vi "CSM_Curve Editor.vi"() -> ()   [LabVIEW 2020, in "Curve Editor.lvlib"]
uses:
  Curve Editor.lvlib
  User Data--cluster.ctl
  <vilib>/Utility/miscctls.llb/LVPointTypeDef.ctl
  7b0969bd-7955-4222-98c9-53128525ee30.vi
  183b1dfd-394f-40bc-8548-5665fe87f6d3.vi
  54737b30-700e-483c-a5e2-87d6bca6278c.vi
  <userlib>/_NEVSTOP/Communicable State Machine(CSM)/AdvanceAPI/CSM - Revert Arguments-Safe String.vi
  <userlib>/_NEVSTOP/Communicable State Machine(CSM)/_Shared/Trim Single-line Text.vi
  <userlib>/_NEVSTOP/Communicable State Machine(CSM)/AdvanceAPI/CSM - Make String Arguments Safe.vi
  <userlib>/_NEVSTOP/Communicable State Machine(CSM)/AdvanceAPI/CSM - Break Down Multiple States String.vi
  <userlib>/_NEVSTOP/Communicable State Machine(CSM)/AdvanceAPI/CSM - Compact Multiple States.vi
  <userlib>/_NEVSTOP/Communicable State Machine(CSM)/AdvanceAPI/CSM - Keywords.vi
  <userlib>/_NEVSTOP/Communicable State Machine(CSM)/addons/API-String-Arugments-Support/_Support/Data To API String Arguments.vi
  <vilib>/Utility/file.llb/Read Delimited Spreadsheet (string).vi
  <userlib>/_NEVSTOP/Communicable State Machine(CSM)/addons/API-String-Arugments-Support/_Support/Convert API String Arguments to Data(variant).vi
  <userlib>/_NEVSTOP/Communicable State Machine(CSM)/Communicable State Machine.lvlib
panel:
  in  "Tab Control":enum32{"Page 1"}(tab)
  in  "动作列表框":i32(listbox) caption="曲线片段"
  in  "循环树形":string(tree) caption="循环编辑"
  in  "打开按钮":bool
  in  "保存按钮":bool
  in  "另存为按钮":bool
  in  "新建按钮":bool
  out "曲线预览":cluster{"X":dbl[], "Y":dbl[]}(graph)
  out "总时长[秒]":dbl format="%.2f"
  out "State History":string
  in  "Name (\"\" to Use UUID)":string="Curve Editor"
  # "曲线编辑"
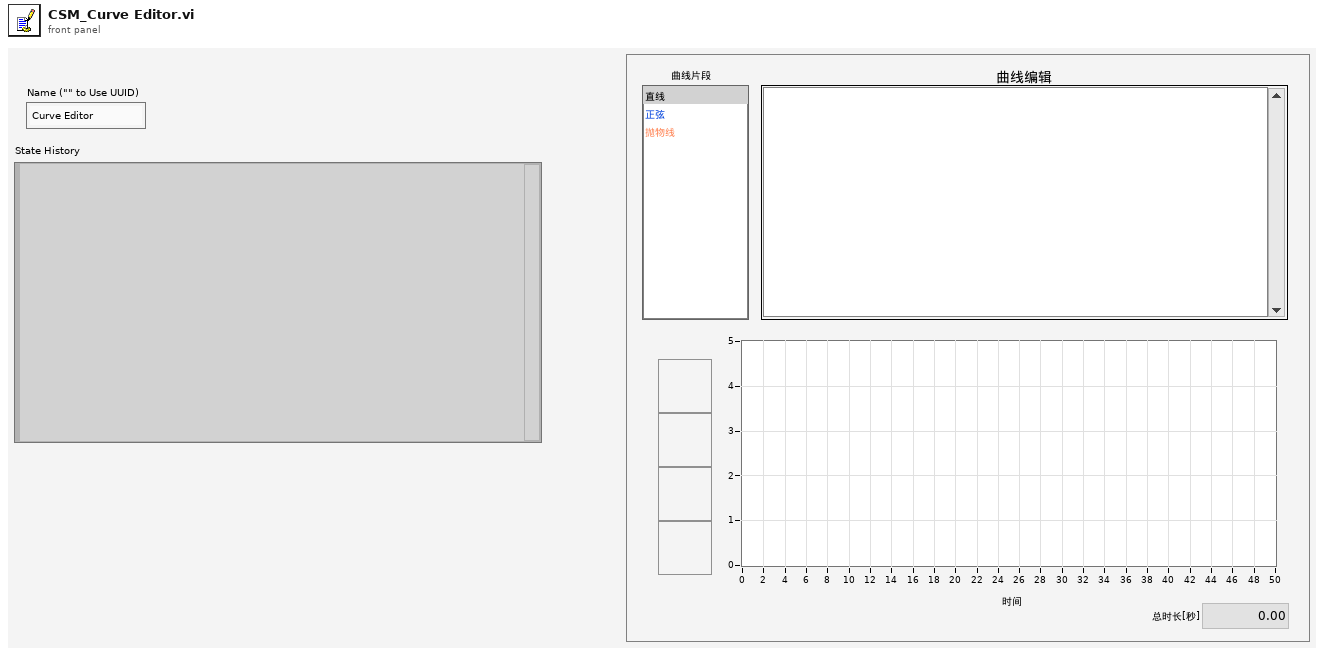
[diagram p1: front panel]
types:
  T1 = enum32{"Invalid", "Standard", "Closed", "Hidden", "Minimized", "Maximized"}
  T2 = enum32{"invalid app kind", "Development System", "Run Time System", "Student Edition", "Embedded LabVIEW", "Evaluation", "Custom"}
  T3 = cluster{"开始路径":path, "默认名称":string, "类型(后缀名)":string, "类型标签":string}
  T4 = typedef "LVPointTypeDef.ctl" = cluster{"Horizontal":i16, "Vertical":i16}
  T5 = enum16{"open", "replace", "create", "open or create", "replace or create", "replace or create with confirmation"}
  T6 = typedef "Communicable State Machine.lvlib/_CSM_Response Source Message.ctl" = cluster{"‘State":string, "’Arguments":string, "’Error":errorcluster}
  T7 = typedef "LVPoint32TypeDef.ctl" = cluster{"Horizontal":i32, "Vertical":i32}
  T8 = typedef "Curve Editor.lvlib/User Data--cluster.ctl" = cluster{"窗体标题":string, "文件参数":cluster{"默认路径":path, "默认名称":string, "类型(后缀名)":string, "类型标签":string}, "颜色符号列表":cluster{"项名":string, "颜色":u32, "符号":i32}[], "循环数组":string[], "文件路径":path, "文件已保存":bool, "存盘提醒":bool}
  T9 = cluster{"Core":cluster{"Current VI Reference":refnum<vi>, "Close Panel on Exit?":bool}, "User Data":T8}
  T10 = cluster{"Current VI Reference":refnum<vi>, "Close Panel on Exit?":bool}
  T11 = cluster{"默认路径":path, "默认名称":string, "类型(后缀名)":string, "类型标签":string}
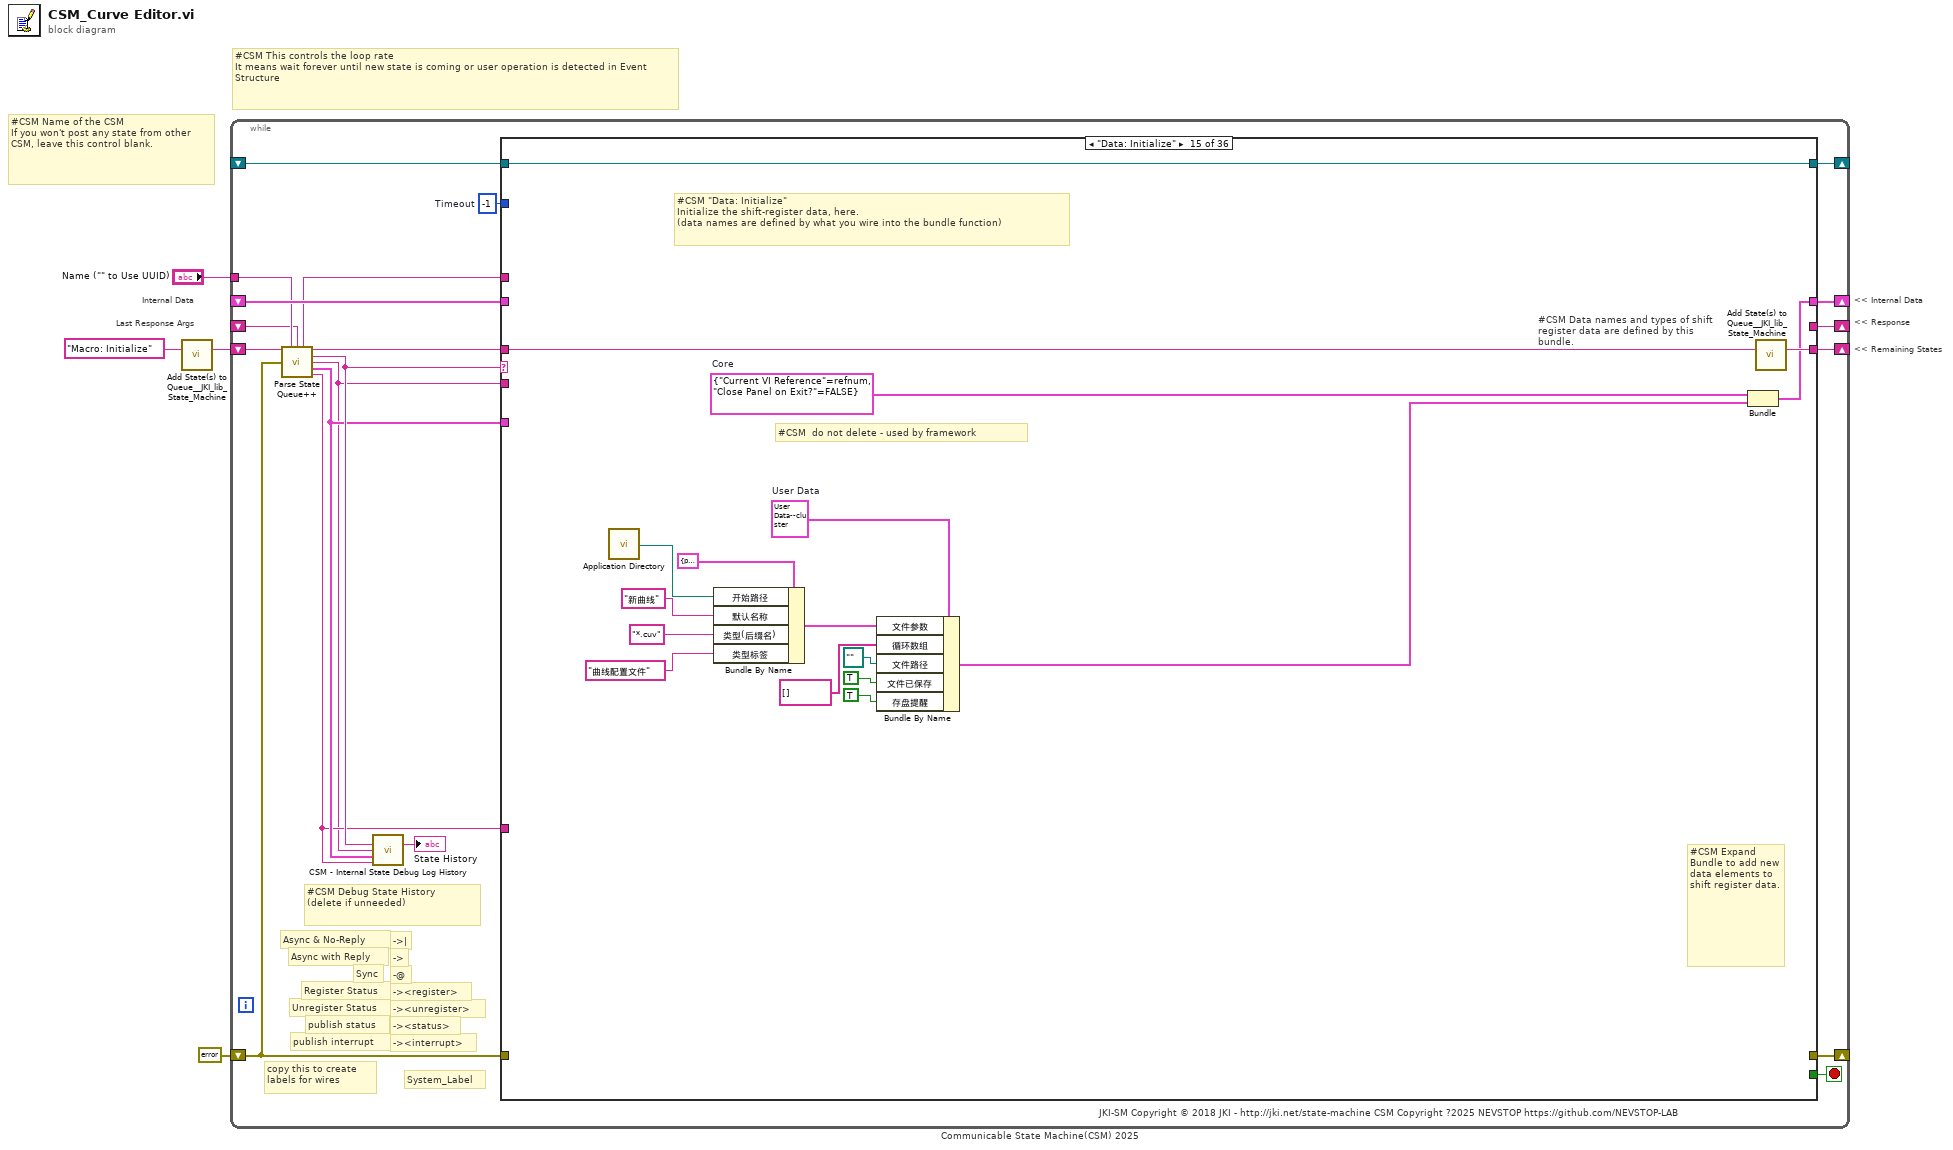
[diagram p0: block diagram]
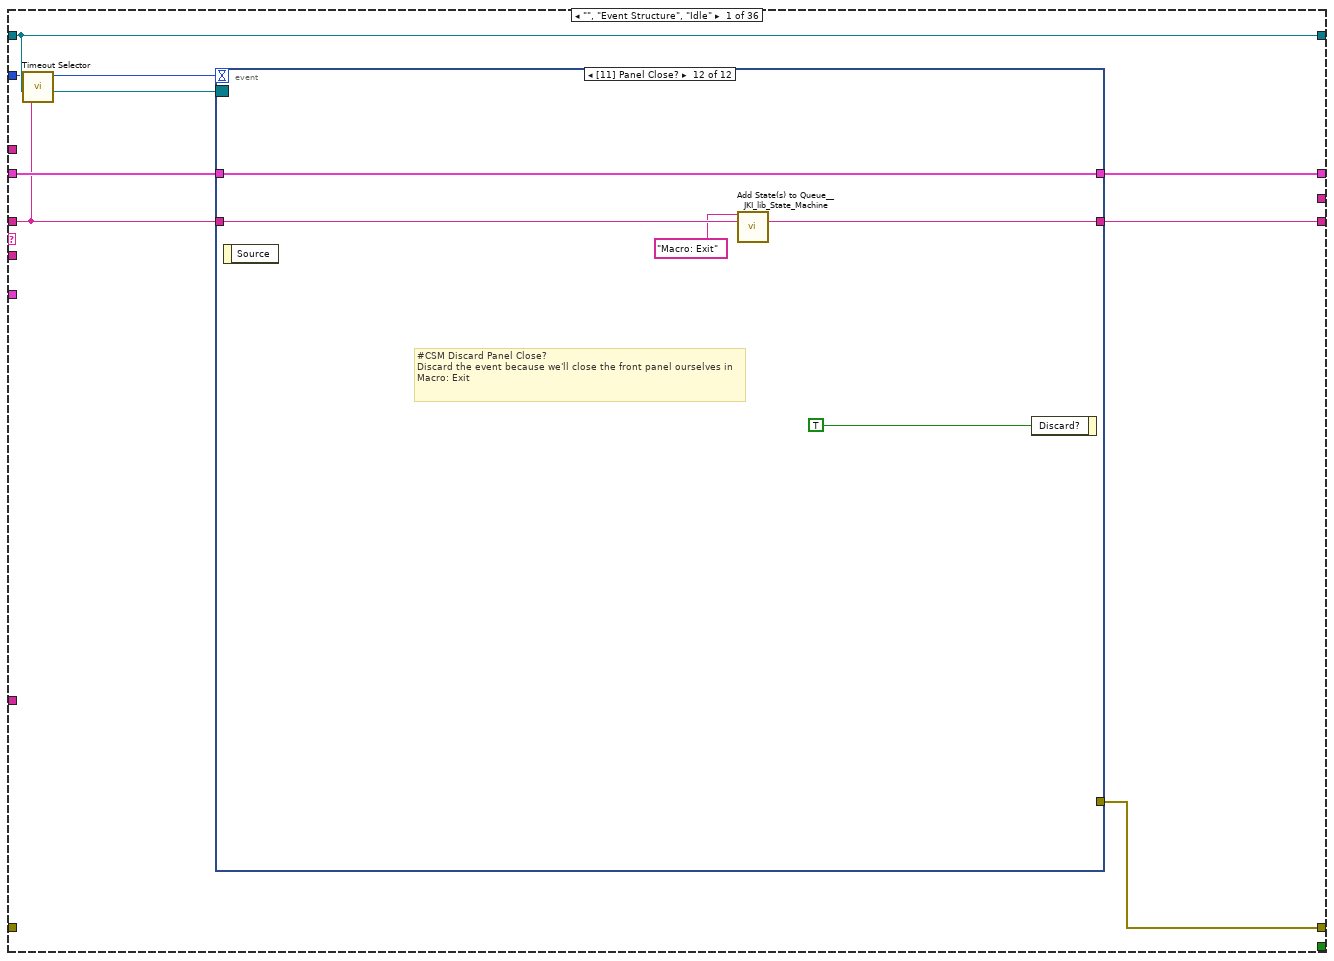
[diagram p2: hidden frame]
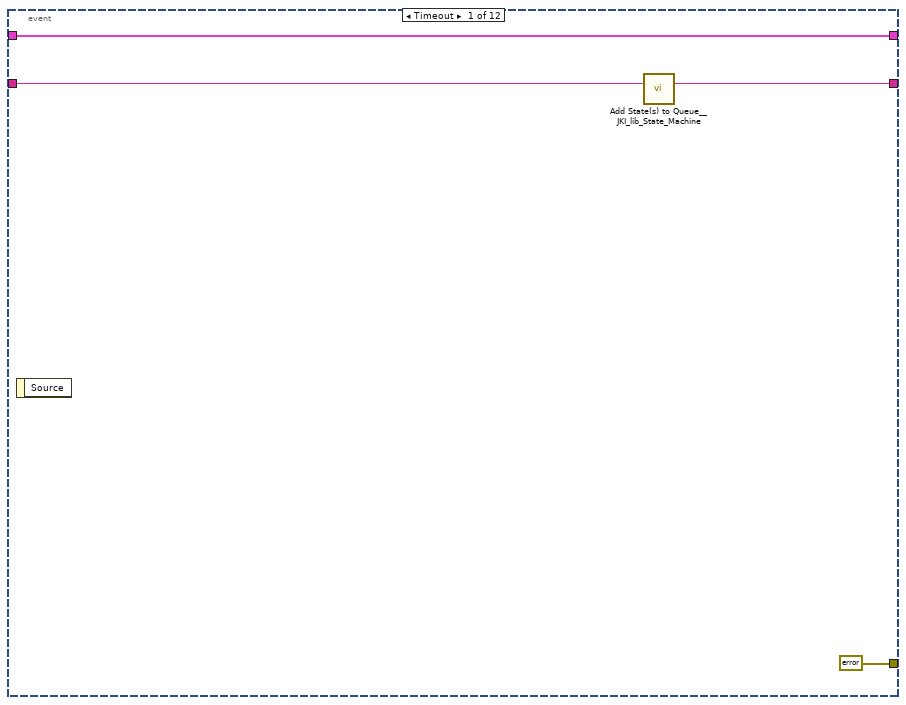
[diagram p3: hidden frame]
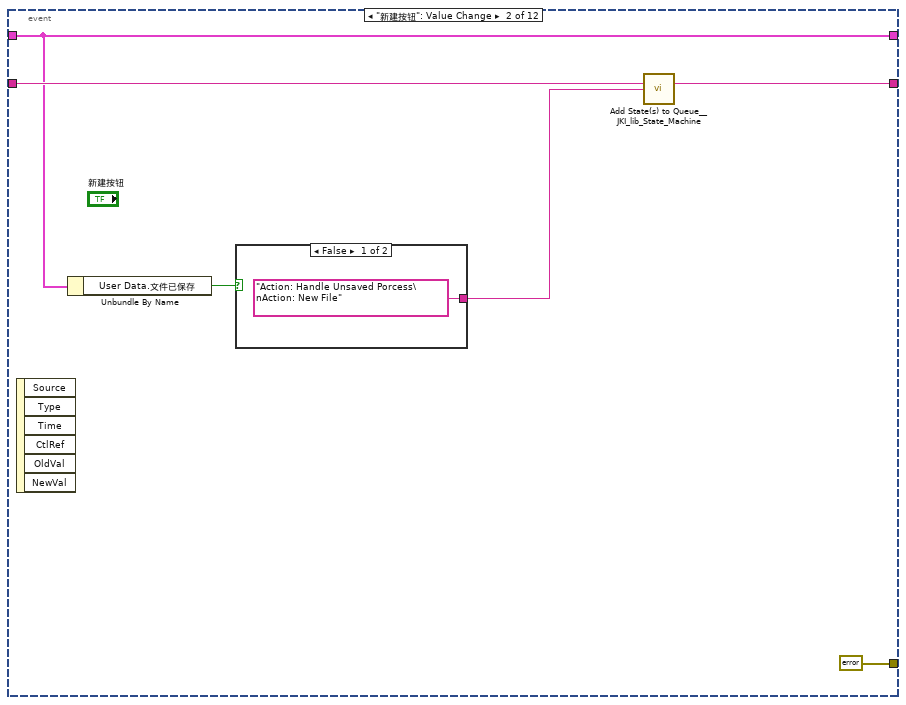
[diagram p4: hidden frame]
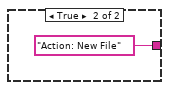
[diagram p5: hidden frame]
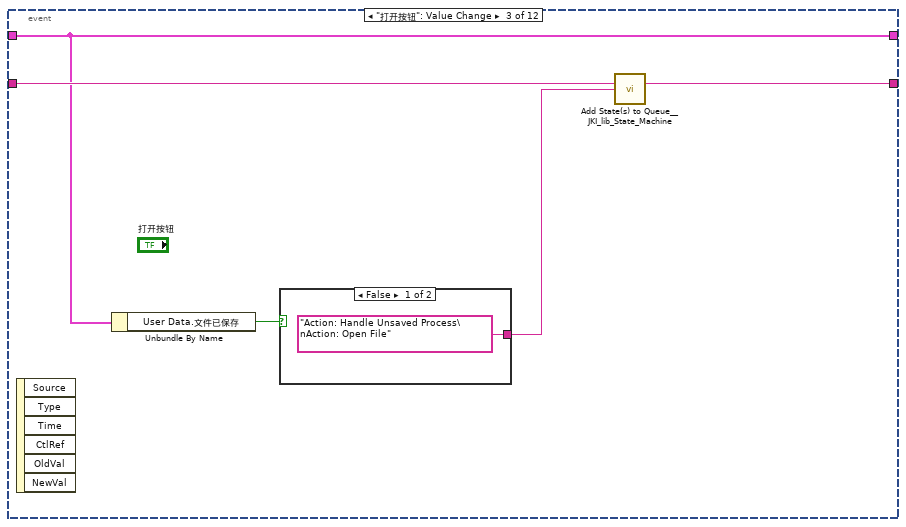
[diagram p6: hidden frame]
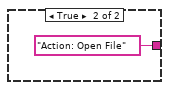
[diagram p7: hidden frame]
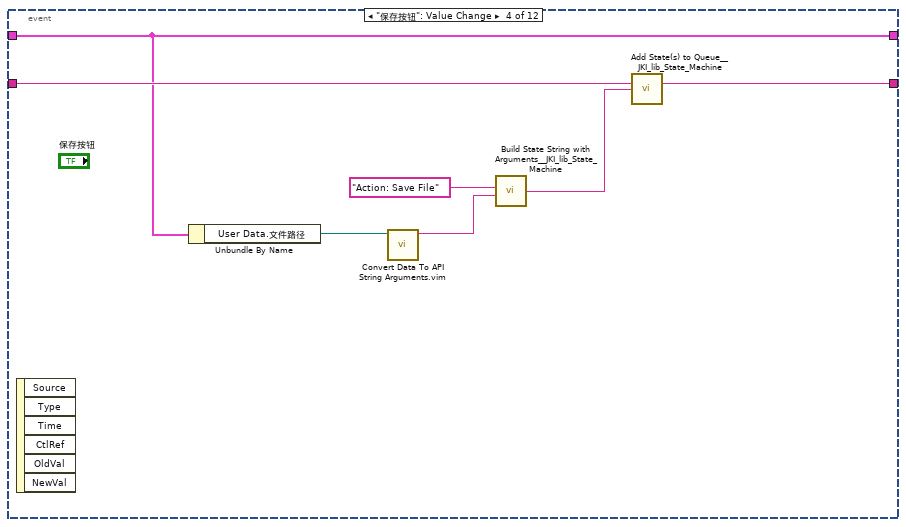
[diagram p8: hidden frame]
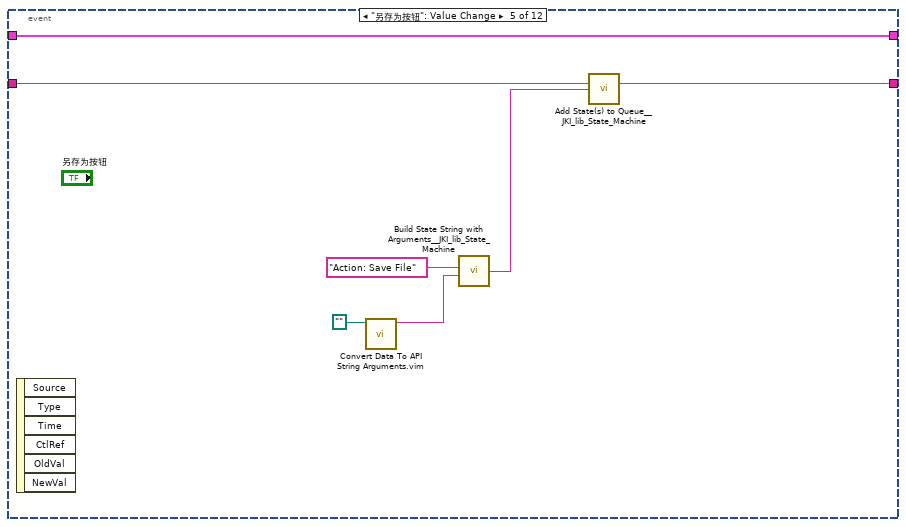
[diagram p9: hidden frame]
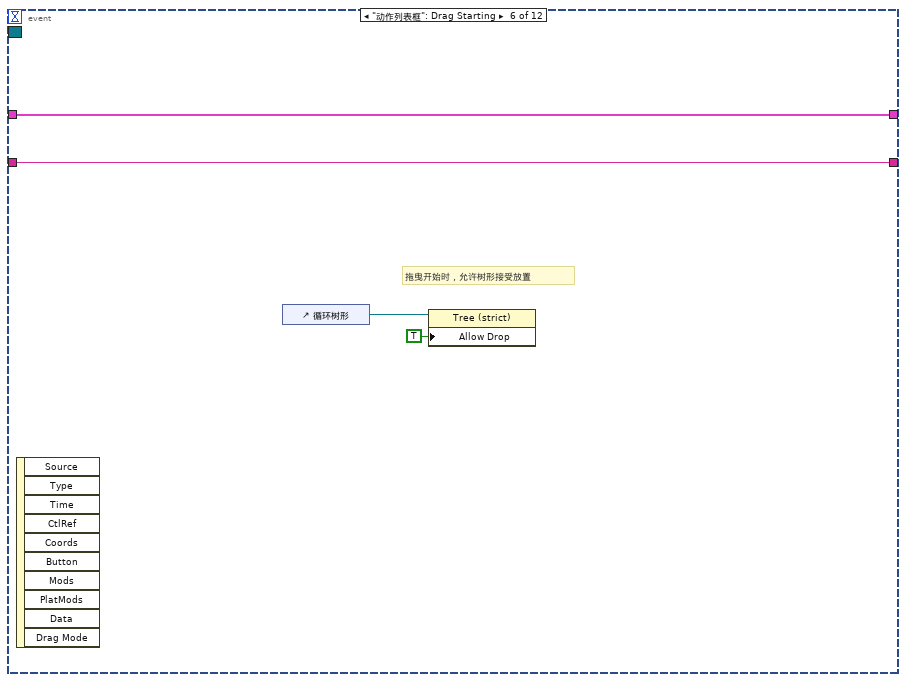
[diagram p10: hidden frame]
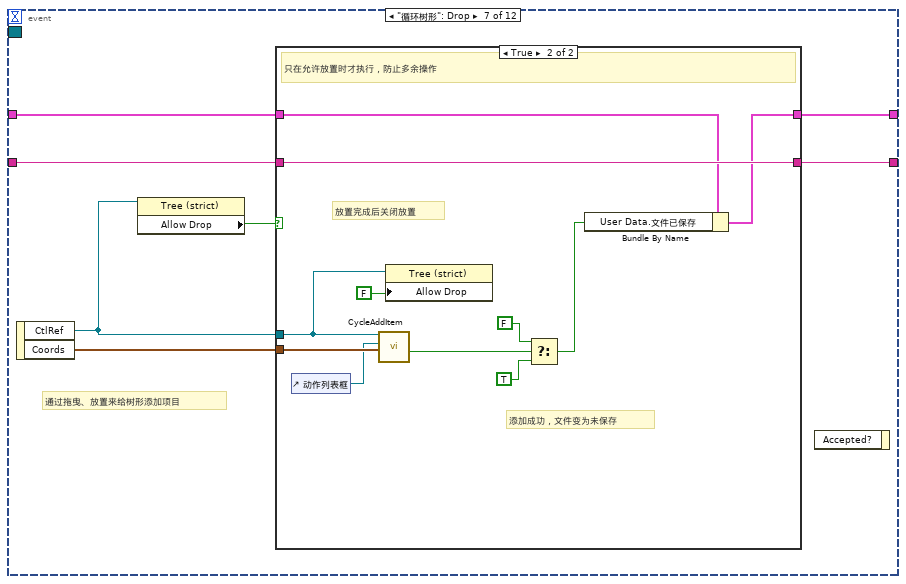
[diagram p11: hidden frame]
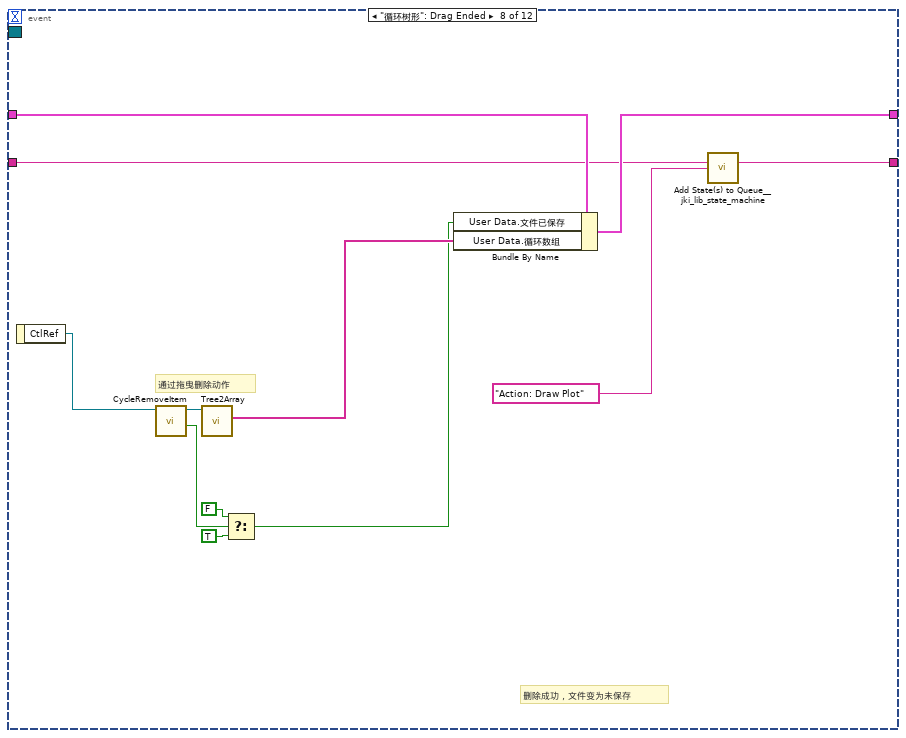
[diagram p13: hidden frame]
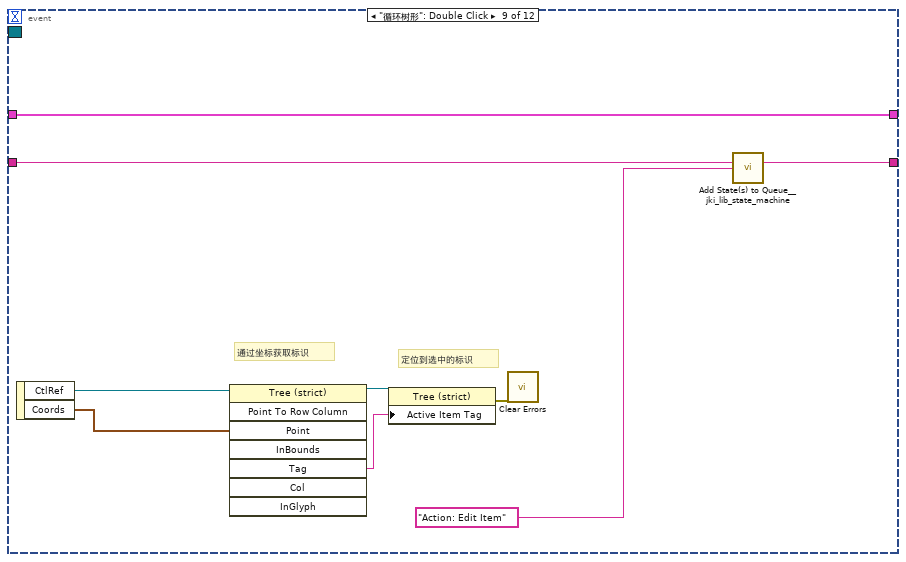
[diagram p14: hidden frame]
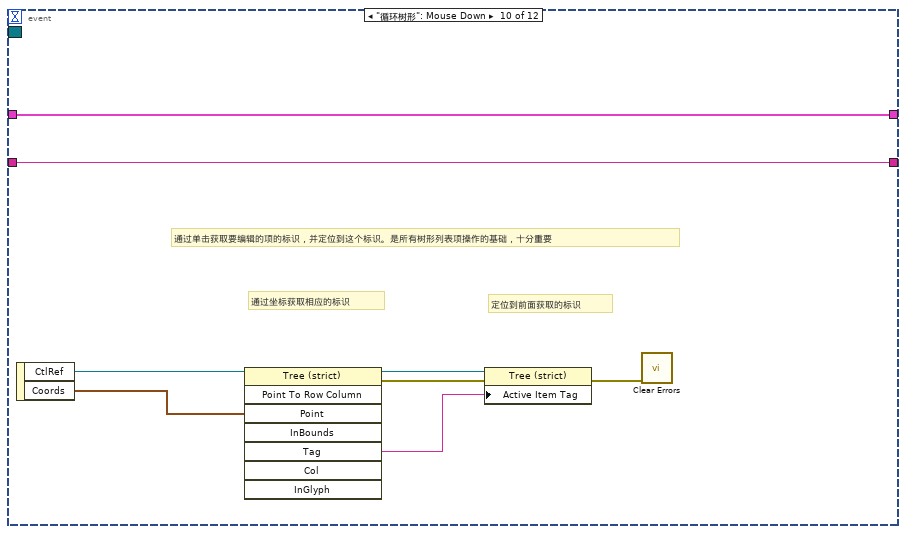
[diagram p15: hidden frame]
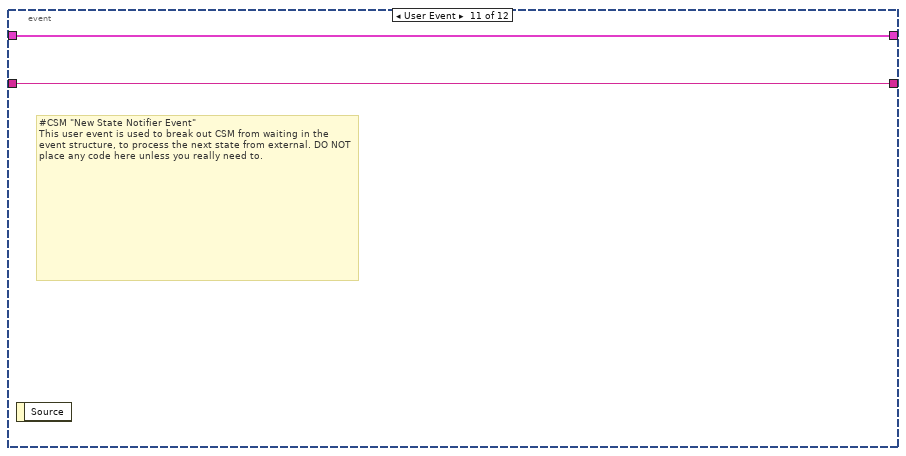
[diagram p16: hidden frame]
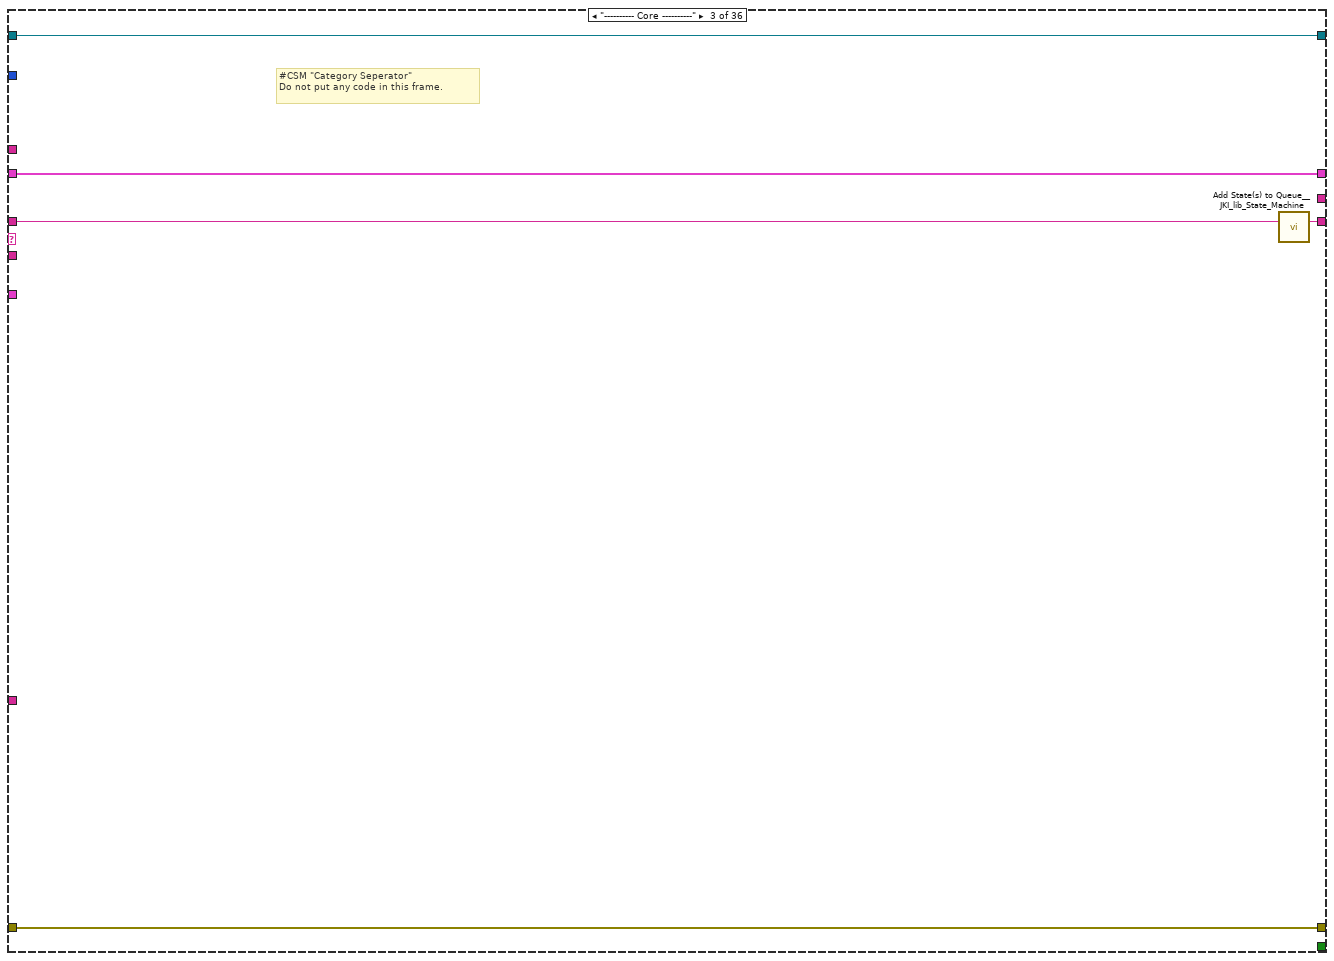
[diagram p18: hidden frame]
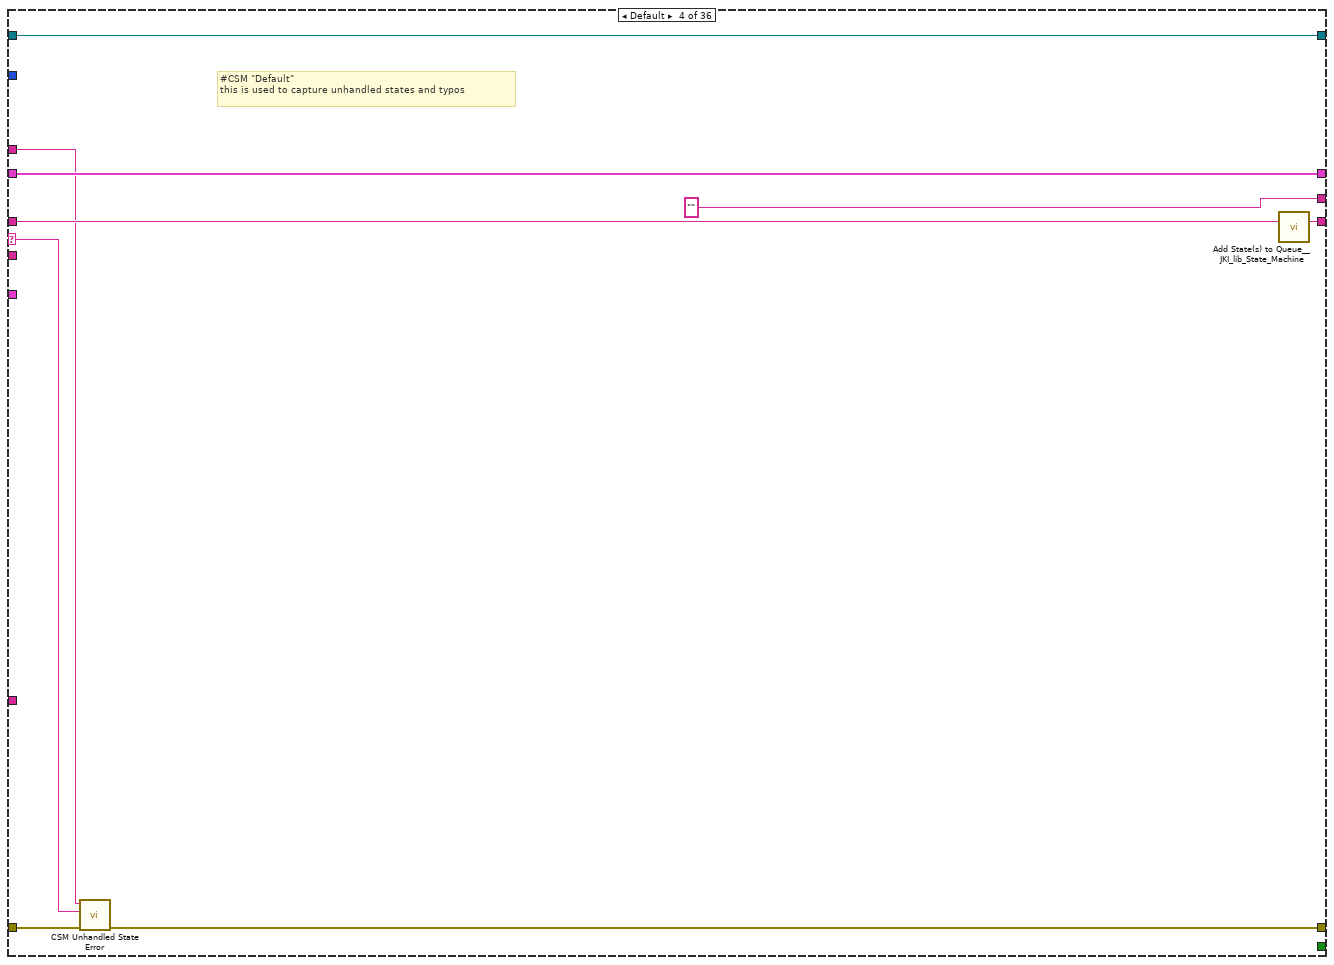
[diagram p19: hidden frame]
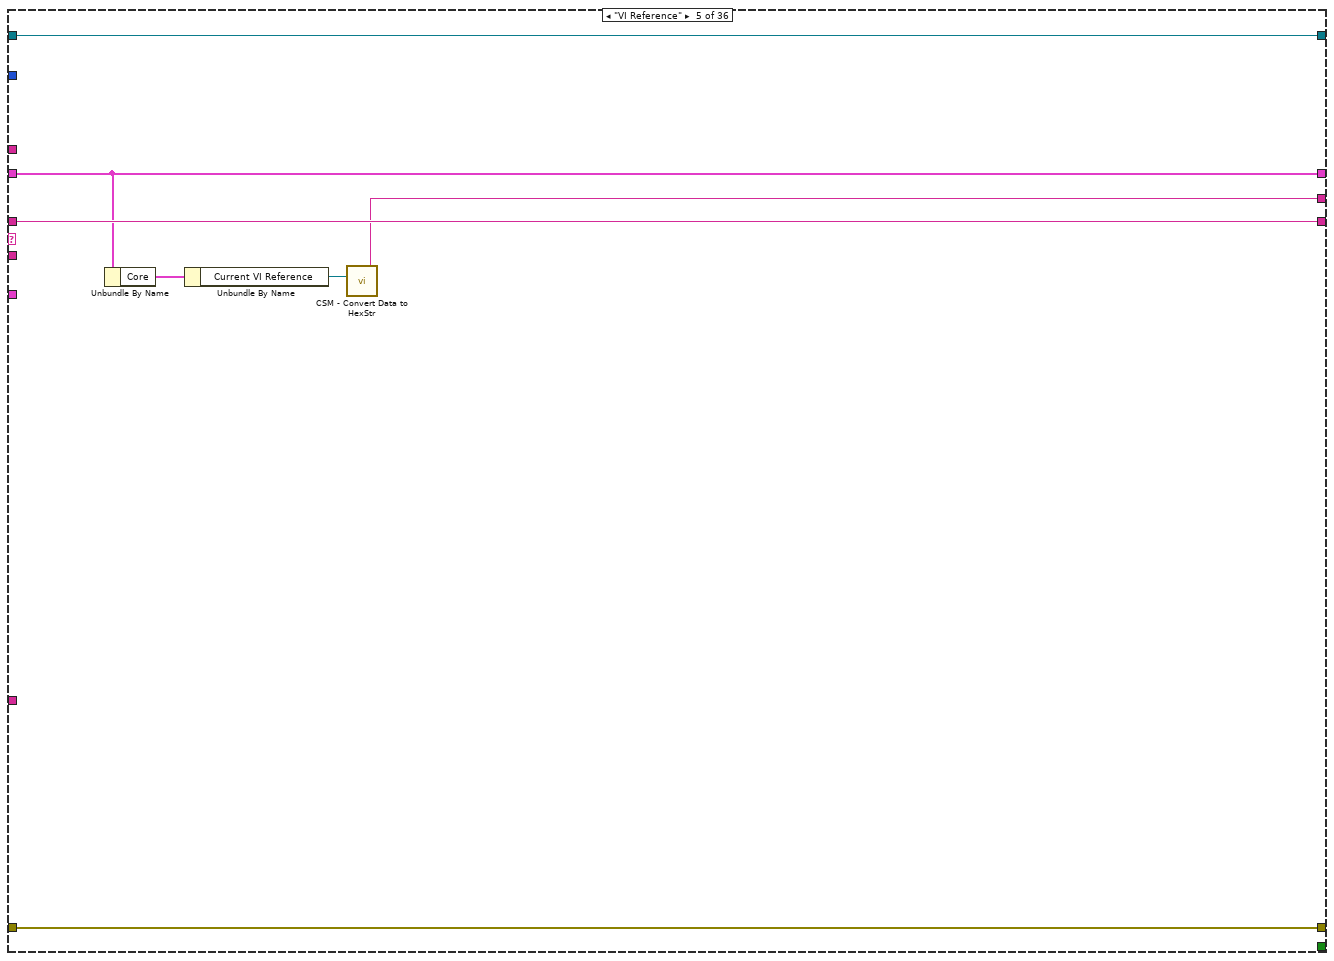
[diagram p20: hidden frame]
diagram:
  # "Last Response Args"
  # "Internal Data"
  # "<< Internal Data"
  # "<< Response"
  # "<< Remaining States"
  # "#CSM Name of the CSM\nIf you won't post any state from other CSM, leave this control blank."
  # "#CSM This controls the loop rate\nIt means wait forever until new state is coming or user operation is detected in Event Structure"
  n1 = call <vilib>:"Add State(s) to Queue__JKI_lib_State_Machine.vi"("State(s) in (\"\")"="Macro: Initialize" ("Init State(\"Macro: Initialize\")")) -> ("States Out"=w1:string)  [unwired: 14 in]
  n2 = while "Communicable State Machine(CSM) 2025" {
    shift-right: [w19] -> _
    shift-left: _ -> [w18]
    shift-right: [w22] -> _
    shift-left: errorcluster {"status"=FALSE, "code"=0, "source"=""} ("error out") -> [w16]
    shift-right: [w21] -> _
    shift-left: w1 -> [w23]
    tunnel: "Name (\"\" to Use UUID)" -> [w12]
    shift-right: [w15] -> _
    shift-left: _ -> [w7]
    shift-right: [w14] -> _
    shift-left: _ -> [w13]
    stop <- w20 stop-if-true
    w17 = -1  # Timeout
    # "#CSM Debug State History\n(delete if unneeded)"
    # "-><interrupt>"
    # "-><status>"
    # "-><unregister>"
    # "-><register>"
    # "-@"
    # "->"
    # "->|"
    # "publish interrupt"
    # "publish status"
    # "Unregister Status"
    # "Register Status"
    # "Sync"
    # "Async with Reply"
    # "Async & No-Reply"
    # "copy this to create labels for wires"
    # "System_Label"
    # "JKI-SM Copyright © 2018 JKI - http://jki.net/state-machine CSM Copyright ?2025 NEVSTOP https://github.com/NEVSTOP-LAB"
    n3 = call <userlib>:"Parse State Queue++.vi"("State Queue"=w23, "Name (\"\" to Use UUID)"=w12, "Response Arguments"=w7, "Previous Error"=w16) -> ("Name Used"=w8:string, "Remaining States"=w24:string, "Current State"=w11:string, "Arguments"=w6:string, "Additional Information"=w10:T6, "Source CSM"=w9:string)  [unwired: 6 in]
    n4 = call <userlib>:"CSM - Internal State Debug Log History.vi"("State"=w11, "Arguments (\"\")"=w6, ">> Response Source Message >>"=w10, "Source (\"\")"=w9) -> ("Debug Log"=→"State History":string)  [unwired: 11 in]
    n5 = case shown="\"Data: Initialize\"" w11 {
      selector: w11 -> [_ _ _ w136 _ _ _ _ _ _ _ _ _ _ _ _ _ _ _ _ _ _ _ _ _ _ _ _ _ _ _ _ _ _ _ _]
      tunnel: w24 -> [w25 w128 w133 w142 w148 w154 w180 w188 w195 w205 w214 w227 w232 w236 w253 w259 w263 w270 w274 w278 w298 w304 w315 w379 w384 w395 w398 w402 w421 w445 w482 w484 w519 w551 w590 w591]
      tunnel: w6 -> [_ _ _ _ _ w152 w176 w183 w191 w199 _ _ _ _ _ _ _ _ _ _ _ w300 w310 _ _ _ _ _ _ _ _ _ _ w548 _ _]
      tunnel: w18 -> [w31 w127 w130 w140 w147 w160 w181 w186 w193 w203 w213 w222 w230 w234 _ w255 w261 w269 w273 w276 w285 w302 w312 w377 w382 w393 w397 w400 w403 w447 w475 w486 w520 w550 w571 w593]
      tunnel: [w30 _ w131 w134 w149 errorcluster {"status"=FALSE, "code"=0, "source"=""} ("error out") w173 w182 w189 w202 _ _ _ _ _ w256 _ w264 w272 _ _ w301 w313 _ _ _ _ _ _ _ w483 w493 w529 w558 _ w603] -> w22
      tunnel: w16 -> [_ _ w131 w135 w149 w158 w174 w184 w190 _ _ _ _ _ _ _ _ _ _ _ _ _ _ _ _ _ _ _ _ _ w483 w493 w529 w558 _ w603]
      tunnel: [w32 w128 w132 w141 w148 w156 w179 w187 w194 w206 w214 w226 w231 w235 w252 w258 w262 w270 w274 w277 w297 w303 w314 w378 w383 w394 w398 w401 w420 w444 w482 w485 w517 w552 w589 w592] -> w21
      tunnel: [_ _ _ _ _ _ TRUE _ _ _ _ _ TRUE _ _ _ _ _ _ _ _ _ _ _ _ _ _ _ _ _ _ _ _ _ _ _] -> w20
      tunnel: [w29 w127 w130 w140 w147 w160 w181 w186 w193 w204 w213 w225 w230 w234 w251 w255 w261 w269 w273 w276 w283 w302 w312 w377 w382 w393 w397 w400 w404 w448 w475 w487 w518 w553 w574 w594] -> w19
      tunnel: w17 -> [w27 _ _ _ _ _ _ _ _ _ _ _ _ _ _ _ _ _ _ _ _ _ _ _ _ _ _ _ _ _ _ _ _ _ _ _]
      tunnel: w9 -> [_ _ _ _ _ w151 _ _ _ w200 _ _ _ _ _ _ _ _ _ _ _ _ _ _ _ _ _ _ _ _ _ _ _ _ _ _]
      tunnel: w10 -> [_ _ _ _ _ w150 _ _ _ w201 _ _ _ _ _ _ _ _ _ _ _ _ _ _ _ _ _ _ _ _ _ _ _ _ _ _]
      tunnel: [_ _ _ "" w143 _ _ _ _ _ _ _ _ _ _ _ _ _ _ _ _ _ _ _ _ _ _ _ _ _ _ _ _ _ _ _] -> w15
      tunnel: [w28 w126 w129 w138 w146 w159 w177 w185 w192 w207 w212 w216 w228 w233 w249 w254 w260 w268 w271 w275 w296 w299 w309 w376 w380 w386 w396 w399 w419 w457 w481 w492 w528 w557 w588 w602] -> w14
      tunnel: w13 -> [w28 w126 w129 w138 w146 w159 w177 w185 w192 w207 w212 w216 w228 w233 w249 w254 w260 _ w271 w275 w296 w299 w309 w376 w380 w386 w396 w399 w419 w457 w481 w492 w528 w557 w588 w602]
      tunnel: w8 -> [_ _ _ w137 _ _ w175 _ _ _ _ _ _ _ _ _ _ w267 _ _ _ _ _ _ _ _ _ _ _ _ _ _ _ _ _ _]
      frame "", "Event Structure", "Idle" {
        n6 = call <userlib>:"Timeout Selector.vi"("Remaining States"=w25, "Timeout Expected"=w27) -> ("Timeout"=w26:i32)  [unwired: 5 in]
        n7 = event shown="[11] Panel Close?" {
          selector: w28 -> [_ _ _ _ _ _ _ _ _ _ _ _]
          dyn-events: _ -> [_ _ _ _ _ _ _ _ _ _ _ _]
          timeout: w26 -> [_ _ _ _ _ _ _ _ _ _ _ _]
          tunnel: w25 -> [w36 w42 w49 w57 w63 w69 w70 w91 w103 w118 w119 w125]
          tunnel: [w35 w41 w48 w58 w64 w69 w71 w92 w104 w118 w119 w124] -> w32
          tunnel: w31 -> [w34 w38 w47 w55 w65 w68 w73 w101 w110 w117 w120 w123]
          tunnel: [errorcluster {"status"=FALSE, "code"=0, "source"=""} ("error out") errorcluster {"status"=FALSE, "code"=0, "source"=""} ("error out") _ _ _ _ _ _ _ _ _ _] -> w30
          tunnel: [w34 w38 w47 w55 w65 w68 w72 w100 w110 w117 w120 w123] -> w29
          event Timeout {
            n8 = event-data() -> ()  [unwired: 1 in, 1 out]
            n9 = call <vilib>:"Add State(s) to Queue__JKI_lib_State_Machine.vi"("State(s) in (\"\")"=w36) -> ("States Out"=w35:string)  [unwired: 14 in]
          }
          event "新建按钮": Value Change {
            n10 = event-data() -> ()  [unwired: 1 in, 6 out]
            n11 = Unbundle By Name(w38) -> ("User Data.文件已保存"=w39:bool)
            n12 = case shown="False" w39 {
              tunnel: ["Action: Handle Unsaved Porcess\nAction: New File" "Action: New File"] -> w37
              frame False {
              }
              frame True {
              }
            }
            n13 = call <vilib>:"Add State(s) to Queue__JKI_lib_State_Machine.vi"("State(s) in (\"\")"=w42, "State(s) at Back (\"\")"=w37) -> ("States Out"=w41:string)  [unwired: 13 in]
          }
          event "打开按钮": Value Change {
            n14 = event-data() -> ()  [unwired: 1 in, 6 out]
            n15 = Unbundle By Name(w47) -> ("User Data.文件已保存"=w46:bool)
            n16 = case shown="False" w46 {
              tunnel: ["Action: Handle Unsaved Process\nAction: Open File" "Action: Open File"] -> w45
              frame False {
              }
              frame True {
              }
            }
            n17 = call <vilib>:"Add State(s) to Queue__JKI_lib_State_Machine.vi"("State(s) in (\"\")"=w49, "State(s) at Back (\"\")"=w45) -> ("States Out"=w48:string)  [unwired: 13 in]
          }
          event "保存按钮": Value Change {
            n18 = event-data() -> ()  [unwired: 1 in, 6 out]
            n19 = Unbundle By Name(w55) -> ("User Data.文件路径"=w54:path)
            n20 = call "Convert Data To API String Arguments.vim"("Data"=w54) -> ("API String"=w53:string)  [unwired: 7 in, 1 out]
            n21 = call <vilib>:"Build State String with Arguments__JKI_lib_State_Machine.vi"("Arguments (\"\")"=w53, "State"="Action: Save File" ("State(s) at Back (\"\")")) -> ("State with Arguments"=w52:string)  [unwired: 4 in]
            n22 = call <vilib>:"Add State(s) to Queue__JKI_lib_State_Machine.vi"("State(s) in (\"\")"=w57, "State(s) at Back (\"\")"=w52) -> ("States Out"=w58:string)  [unwired: 13 in]
          }
          event "另存为按钮": Value Change {
            n23 = event-data() -> ()  [unwired: 1 in, 6 out]
            n24 = call "Convert Data To API String Arguments.vim"("Data"=path "") -> ("API String"=w59:string)  [unwired: 7 in, 1 out]
            n25 = call <vilib>:"Build State String with Arguments__JKI_lib_State_Machine.vi"("Arguments (\"\")"=w59, "State"="Action: Save File" ("State(s) at Back (\"\")")) -> ("State with Arguments"=w61:string)  [unwired: 4 in]
            n26 = call <vilib>:"Add State(s) to Queue__JKI_lib_State_Machine.vi"("State(s) in (\"\")"=w63, "State(s) at Back (\"\")"=w61) -> ("States Out"=w64:string)  [unwired: 13 in]
          }
          event "动作列表框": Drag Starting {
            # "拖曳开始时，允许树形接受放置"
            n27 = event-data() -> ()  [unwired: 1 in, 10 out]
            n28 = control-ref of="循环树形"() -> (w66:refnum<vi>)
            n29 = property class="Tree (strict)"(reference=w66, "Allow Drop"=TRUE ("拖曳/放置:允许放置")) -> ()  [unwired: 1 in, 2 out]
          }
          event "循环树形": Drop {
            # "通过拖曳、放置来给树形添加项目"
            n30 = event-data() -> ("CtlRef"=w75:refnum<vi>, "Coords"=w74:T7)  [unwired: 1 in]
            n31 = property class="Tree (strict)"(reference=w75) -> ("Allow Drop"=w76:bool)  [unwired: 1 in, 2 out]
            n32 = case shown="True" w76 {
              tunnel: w74 -> [_ w89]
              tunnel: w75 -> [_ w86]
              tunnel: w73 -> [w78 w81]
              tunnel: [w78 w79] -> w72
              tunnel: [w77 w82] -> w71
              tunnel: w70 -> [w77 w82]
              frame False {
              }
              frame True {
                # "添加成功，文件变为未保存"
                # "放置完成后关闭放置"
                # "只在允许放置时才执行，防止多余操作"
                n33 = control-ref of="动作列表框"() -> (w88:refnum<vi>)
                n34 = call "CycleAddItem.vi"("Coords"=w89, "动作列表框"=w88, "TreeControl输入"=w86) -> ("添加成功"=w83:bool)  [unwired: 6 in, 2 out]
                n35 = property class="Tree (strict)"(reference=w86, "Allow Drop"=FALSE ("拖曳/放置:允许放置")) -> ()  [unwired: 1 in, 2 out]
                n36 = Select(t=FALSE, s=w83, f=TRUE) -> (s? t:f=w80:bool)
                n37 = Bundle By Name(cluster=w81, "User Data.文件已保存"=w80) -> (w79:T9)
              }
            }
            n38 = event-data() -> ()  [unwired: 2 in, 1 out]
          }
          event "循环树形": Drag Ended {
            # "删除成功，文件变为未保存"
            # "通过拖曳删除动作"
            n39 = event-data() -> ("CtlRef"=w95:refnum<vi>)  [unwired: 1 in]
            n40 = call "CycleRemoveItem.vi"("TreeControl输入"=w95) -> ("删除成功"=w98:bool, "TreeControl输出"=w99:refnum<vi>)  [unwired: 8 in, 1 out]
            n41 = call "Tree2Array.vi"("TreeControl输入"=w99) -> ("循环数组"=w94:string[])  [unwired: 9 in, 1 out]
            n42 = Select(t=FALSE, s=w98, f=TRUE) -> (s? t:f=w93:bool)
            n43 = Bundle By Name(cluster=w101, "User Data.文件已保存"=w93, "User Data.循环数组"=w94) -> (w100:T9)
            n44 = call <vilib>:"Add State(s) to Queue__jki_lib_state_machine.vi"("State(s) in (\"\")"=w91, "State(s) at Back (\"\")"="Action: Draw Plot" ("State(s) at Back (\"\")")) -> ("States Out"=w92:string)  [unwired: 13 in]
          }
          event "循环树形": Double Click {
            # "定位到选中的标识"
            # "通过坐标获取标识"
            n45 = event-data() -> ("CtlRef"=w105:refnum<vi>, "Coords"=w106:T7)  [unwired: 1 in]
            n46 = invoke class="Tree (strict)" method="Point To Row Column"(reference=w105, "Point"=w106) -> (reference out=w107:refnum<vi>, "Tag"=w108:string)  [unwired: 6 in, 6 out]
            n47 = property class="Tree (strict)"(reference=w107, "Active Item Tag"=w108) -> (error out=w109:errorcluster)  [unwired: 1 in, 1 out]
            n48 = call <vilib>:"Clear Errors.vi"("error in (no error)"=w109) -> ()  [unwired: 5 in, 2 out]
            n49 = call <vilib>:"Add State(s) to Queue__jki_lib_state_machine.vi"("State(s) in (\"\")"=w103, "State(s) at Back (\"\")"="Action: Edit Item" ("State(s) at Back (\"\")")) -> ("States Out"=w104:string)  [unwired: 13 in]
          }
          event "循环树形": Mouse Down {
            # "定位到前面获取的标识"
            # "通过坐标获取相应的标识"
            # "通过单击获取要编辑的项的标识，并定位到这个标识。是所有树形列表项操作的基础，十分重要"
            n50 = event-data() -> ("CtlRef"=w112:refnum<vi>, "Coords"=w111:T7)  [unwired: 1 in]
            n51 = invoke class="Tree (strict)" method="Point To Row Column"(reference=w112, "Point"=w111) -> (reference out=w113:refnum<vi>, error out=w115:errorcluster, "Tag"=w114:string)  [unwired: 6 in, 5 out]
            n52 = property class="Tree (strict)"(reference=w113, error in=w115, "Active Item Tag"=w114) -> (error out=w116:errorcluster)  [unwired: 1 out]
            n53 = call <vilib>:"Clear Errors.vi"("error in (no error)"=w116) -> ()  [unwired: 5 in, 2 out]
          }
          event User Event {
            # "#CSM \"New State Notifier Event\"\nThis user event is used to break out CSM from waiting in the event structure, to process the next state from external. DO NOT place any code here unless you really need to."
            n54 = event-data() -> ()  [unwired: 1 in, 1 out]
          }
          event Panel Close? {
            # "#CSM Discard Panel Close?\nDiscard the event because we'll close the front panel ourselves in Macro: Exit"
            n55 = event-data() -> ()  [unwired: 1 in, 1 out]
            n56 = call <vilib>:"Add State(s) to Queue__JKI_lib_State_Machine.vi"("State(s) in Front (\"\")"="Macro: Exit", "State(s) in (\"\")"=w125) -> ("States Out"=w124:string)  [unwired: 13 in]
            n57 = event-data("Discard?"=TRUE) -> ()  [unwired: 1 in, 1 out]
          }
        }
      }
      frame "CSM Documentation" {
        # "#CSM State Syntax\n\n// Comment line, all text to the right of “//” will be ignored\n// Local Message Example\nDoSth: DoA >> Arguments\n\n// Sync Call Example\nAPI: xxxx >> Arguments -@ TargetModule\n\n// Async Call Example\nAPI: xxxx >> Arguments -> TargetModule\n\n// Async Call without Reply Example\nAPI: xxxx >> Arguments ->| TargetModule\n\n// Broadcast normal status:\nStatus >> StatusArguments  -><status>\n\n// Broadcast Interrupt status:\nInterrupt >> StatusArguments  -><interrupt>\n\n// Register Source Module's status to Handler Module\nStatus@Source Module >> Handler Module@Handler Module -><register>\n\n// Unegister Source Module's status\nStatus@Source Module >> Handler Module -><unregister>"
        # "#CSM README FIRST\n\nCommunicable State Machine(CSM) is a LabVIEW application framework that builds upon JKI State Machine(JKISM). It follows the pattern of JKISM and extends the keywords to describe message communication between modules, including concepts such as Sync-Message, Async-Message, Subscription/Unsubscription of status - essential elements for creating reusable code modules. For more information, please visit the CSM wiki: https://nevstop-lab.github.io/CSM-Wiki/\n\nFor instructions on JKI State Machine, visit: \n    http://jki.net/state-machine/\nFor information about CSM, visit: \n    https://github.com/NEVSTOP-LAB"
        # "#CSM \"Documentation\"\nCase for holding CSM Documenation"
      }
      frame "---------- Core ----------" {
        # "#CSM \"Category Seperator\"\nDo not put any code in this frame."
        n58 = call <vilib>:"Add State(s) to Queue__JKI_lib_State_Machine.vi"("State(s) in (\"\")"=w133) -> ("States Out"=w132:string)  [unwired: 14 in]
      }
      frame Default {
        # "#CSM \"Default\"\nthis is used to capture unhandled states and typos"
        n59 = call <userlib>:"CSM Unhandled State Error.vi"("error in (no error)"=w135, "Undefined State"=w136, "CSM Name"=w137) -> ("error out"=w134:errorcluster)  [unwired: 8 in]
        n60 = call <vilib>:"Add State(s) to Queue__JKI_lib_State_Machine.vi"("State(s) in (\"\")"=w142) -> ("States Out"=w141:string)  [unwired: 14 in]
      }
      frame "VI Reference" {
        n61 = Unbundle By Name(w147) -> ("Core"=w145:T10)
        n62 = Unbundle By Name(w145) -> ("Current VI Reference"=w144:refnum<vi>)
        n63 = call <userlib>:"CSM - Convert Data to HexStr.vi"("Variant"=w144) -> ("HEX String (0-9,A-F)"=w143:string)  [unwired: 8 in]
      }
      frame "Error Handler" {
        # "#CSM Disable this error dialog if you need"
        # "#CSM \"Error Handler\"\nYou can also output any states to clean-up after errors occur"
        # "Clear error"
        n64 = case shown="Error" w158 {
          selector: w158 -> [_ w167]
          tunnel: [w165 w169] -> w155
          tunnel: w154 -> [w165 w168]
          tunnel: [w164 w167] -> w153
          tunnel: w152 -> [w166 _]
          tunnel: w151 -> [_ _]
          tunnel: w150 -> [_ _]
          frame No Error {
            n65 = call <userlib>:"CSM - Convert Argument to Error.vi"("Argument"=w166) -> ("Error"=w164:errorcluster)  [unwired: 4 in]
            n66 = flat-sequence {
              frame #0 {
                # "#CSM External Error Handler Case\nUsually, it's because This CSM register others' \"Error Occurred\" status with \"Error Handler\". If other CSM have any error, the error will be passed here for central handling."
              }
            }
          }
          frame Error {
            # "#CSM Internal Error Handler Case \nIf any error Occurred, \"Error Occurred\" \nstatus update will be broadcasted to system.\nParameter is Error Cluster."
            n67 = call <userlib>:"CSM - Convert Error to Argument.vi"("Error"=w167) -> ("Argument"=w171:string)  [unwired: 4 in]
            n68 = call <vilib>:"Build State String with Arguments__JKI_lib_State_Machine.vi"("Arguments (\"\")"=w171, "State"="Error Occurred" ("Status with Arguments")) -> ("State with Arguments"=w170:string)  [unwired: 4 in]
            n69 = call <userlib>:"CSM - Broadcast Status Change.vi"("Status With Arguments"=w170, "State Queue"=w168) -> ("Remaining States"=w169:string)  [unwired: 13 in]
          }
        }
        n70 = disable-structure shown="Enabled" {
          disable-tunnel: w153 -> [w162 w163]
          frame Enabled {
            # "Unhandled Error -- Display it"
            n71 = call <vilib>:"General Error Handler.vi"("error in (no error)"=w162) -> ()  [unwired: 10 in, 5 out]
          }
          frame Disabled {
            n72 = call <vilib>:"Clear Errors.vi"("error in (no error)"=w163) -> ()  [unwired: 5 in, 2 out]
          }
        }
        n73 = call <vilib>:"Add State(s) to Queue__JKI_lib_State_Machine.vi"("State(s) in Front (\"\")"="// Post Error States", "State(s) in (\"\")"=w155) -> ("States Out"=w156:string)  [unwired: 13 in]
      }
      frame "Critical Error" {
        # "#CSM \"Critical Error\"\nWhen any un-recoverable error occurs, CSM goes into this case."
        # "#CSM Stop in Critical Error\nWhen Critical Error occurs, Stop the loop immediately. Do NOT change this unless you fully understand the impact."
        n74 = call <userlib>:"CSM Critical Error.vi"("error in (no error)"=w174, "Arugments (As Reason)"=w176, "CSM Name"=w175) -> ("error out"=w173:errorcluster)  [unwired: 8 in]
        n75 = call <vilib>:"Add State(s) to Queue__JKI_lib_State_Machine.vi"("State(s) in (\"\")"=w180) -> ("States Out"=w179:string)  [unwired: 14 in]
      }
      frame "Target Timeout Error" {
        # "#CSM \"Target Timeout Error\"\nWhen This CSM could not get the sync-call response in time, This CSM goes into this case."
        n76 = call <userlib>:"CSM Target Timeout Error.vi"("error in (no error)"=w184, "Arguments (As CSM Name)"=w183) -> ("error out"=w182:errorcluster)  [unwired: 9 in]
        n77 = call <vilib>:"Add State(s) to Queue__JKI_lib_State_Machine.vi"("State(s) in (\"\")"=w188) -> ("States Out"=w187:string)  [unwired: 14 in]
      }
      frame "Target Error" {
        # "#CSM \"Target Error\"\nWhen This CSM try to communicate with an un-existed CSM, This CSM goes into this case."
        n78 = call <userlib>:"CSM Target Error.vi"("error in (no error)"=w190, "Arguments (As CSM Name)"=w191) -> ("error out"=w189:errorcluster)  [unwired: 9 in]
        n79 = call <vilib>:"Add State(s) to Queue__JKI_lib_State_Machine.vi"("State(s) in (\"\")"=w195) -> ("States Out"=w194:string)  [unwired: 14 in]
      }
      frame "Async Response", "Response" {
        # "#CSM \"Async Response\"\nHandle Async-call Response (\"Async Response\" for ->)"
        # "#CSM \"Response\"\nHandle Sync-call Response (\"Response\" for -@)"
        n80 = Unbundle(w201) -> ("‘State"=w198:string, "’Arguments"=w197:string, "’Error"=w196:errorcluster)
        n81 = case shown="Default" w198 {
          tunnel: [w208] -> w206
          tunnel: w205 -> [w209]
          tunnel: [w211] -> w204
          tunnel: w203 -> [w211]
          tunnel: [w210] -> w202
          tunnel: w196 -> [w210]
          tunnel: w200 -> [_]
          tunnel: w199 -> [_]
          tunnel: w197 -> [_]
          frame Default {
            # "#CSM Response Comments\nAfter Message is executed, CSM goes to this state for receive the response.\n    For Async Message(->), \"Async Response\" is used. This CSM will goes to \"Async Message Posted\" immediately and receive the \"Async Response\" after the callee finishes the message.\n    For Sync Message(@),  This CSM will wait until the message is done and immediately goes to \"Response\""
            n82 = call <vilib>:"Add State(s) to Queue__JKI_lib_State_Machine.vi"("State(s) in (\"\")"=w209) -> ("States Out"=w208:string)  [unwired: 14 in]
          }
        }
      }
      frame "Async Message Posted" {
        # "#CSM \"Async Message Posted\"\nAfter Async Message is posted (-> or ->| ), CSM goes to this state for post-action.\nYou can use Argument - State to tell which Async Message is called."
      }
      frame "Initialize Core Data" {
        # "#CSM \"Initialize Core Data\"\nThis is used to determine panel behavior on exit"
        # "originally closed?"
        # "exe?"
        # "If panel starts closed or is an EXE, then close it when we exit"
        n83 = property class="VI"() -> ("FP.State"=w219:T1)  [unwired: 2 in, 2 out]
        n84 = control-ref of="Current VI Reference"() -> (w220:refnum<vi>)
        n85 = property class="App"() -> ("App.Kind"=w224:T2)  [unwired: 2 in, 2 out]
        n86 = Equal?(x=w219, y=T1."Closed" ("Front Panel Window:State")) -> (x = y?=w217:bool)
        n87 = Equal?(x=w224, y=T2."Run Time System" ("Application:Kind")) -> ()  [unwired: 1 out]
        n88 = Or(x=w217, y=TRUE) -> (x .or. y?=w221:bool)
        n89 = Bundle By Name(cluster=w222, "Core.Current VI Reference"=w220, "Core.Close Panel on Exit?"=w221) -> (w225:T9)
        n90 = call <vilib>:"Add State(s) to Queue__JKI_lib_State_Machine.vi"("State(s) in (\"\")"=w227) -> ("States Out"=w226:string)  [unwired: 14 in]
      }
      frame "Exit" {
        # "#CSM \"Exit\"\nCase for exiting the loop. No errors that occur here will be handled."
        n91 = call <vilib>:"Add State(s) to Queue__JKI_lib_State_Machine.vi"("State(s) in (\"\")"=w232) -> ("States Out"=w231:string)  [unwired: 14 in]
      }
      frame "---------- Data ----------" {
        # "#CSM \"Category Seperator\"\nDo not put any code in this frame."
        n92 = call <vilib>:"Add State(s) to Queue__JKI_lib_State_Machine.vi"("State(s) in (\"\")"=w236) -> ("States Out"=w235:string)  [unwired: 14 in]
      }
      frame "Data: Initialize" {
        w248 = T8 {"窗体标题"="", "文件参数"={"默认路径"=path "", "默认名称"="", "类型(后缀名)"="", "类型标签"=""}, "颜色符号列表"=[], "循环数组"=[], "文件路径"=path "", "文件已保存"=FALSE, "存盘提醒"=FALSE}  # User Data
        w250 = T10 {"Current VI Reference"=refnum, "Close Panel on Exit?"=FALSE}  # Core
        # "#CSM  do not delete - used by framework"
        # "#CSM Expand Bundle to add new data elements to shift register data."
        # "#CSM Data names and types of shift register data are defined by this bundle."
        # "#CSM \"Data: Initialize\"\nInitialize the shift-register data, here.\n(data names are defined by what you wire into the bundle function)"
        n93 = call <vilib>:"Application Directory.vi"() -> ("Application Directory"=w237:path)
        n94 = Bundle By Name(cluster=T3 {"开始路径"=path "", "默认名称"="", "类型(后缀名)"="", "类型标签"=""} ("文件参数"), "开始路径"=w237, "默认名称"="新曲线" ("文件_默认文件名"), "类型(后缀名)"="*.cuv" ("文件_后缀名"), "类型标签"="曲线配置文件" ("文件_类型标签")) -> (w242:T3)
        n95 = Bundle By Name(cluster=w248, "文件参数"=w242, "循环数组"=string[] [], "文件路径"=path "", "文件已保存"=TRUE, "存盘提醒"=TRUE) -> (w247:T8)
        n96 = Bundle("Core"=w250, "User Data"=w247) -> (w251:T9)  [unwired: 1 in]
        n97 = call <vilib>:"Add State(s) to Queue__JKI_lib_State_Machine.vi"("State(s) in (\"\")"=w253) -> ("States Out"=w252:string)  [unwired: 14 in]
      }
      frame "Data: Cleanup" {
        # "#CSM \"Data: Cleanup\"\nCleanup any data and references, here.\n(this is called automatically, by the Macro: Exit)"
        n98 = Unbundle By Name(w255) -> ("Core.Current VI Reference"=w257:refnum<vi>)
        n99 = Close Reference(reference=w257) -> (error out=w256:errorcluster)  [unwired: 1 in]
        n100 = call <vilib>:"Add State(s) to Queue__JKI_lib_State_Machine.vi"("State(s) in (\"\")"=w259) -> ("States Out"=w258:string)  [unwired: 14 in]
      }
      frame "---------- Events ----------" {
        # "#CSM \"Category Seperator\"\nDo not put any code in this frame."
        n101 = call <vilib>:"Add State(s) to Queue__JKI_lib_State_Machine.vi"("State(s) in (\"\")"=w263) -> ("States Out"=w262:string)  [unwired: 14 in]
      }
      frame "Events: Register" {
        # "#CSM \"Events: Register\"\nRegister user event. New Message Event is registered to break CSM waiting in event structure by default."
        # "#CSM Register New Message Event\nRegister message event to break Waiting in Event structure."
        n102 = call <userlib>:"CSM - Get New State Notifier Event.vi"("Name (\"\" to Use UUID)"=w267) -> ("error out"=w265:errorcluster, "New State Notifier Event"=w266:refnum<user-event>)  [unwired: 9 in]
        n103 = register-events(error in=w265, w266) -> (reference out=w268:refnum<event-registration>, error out=w264:errorcluster)  [unwired: 1 in]
      }
      frame "Events: Unregister" {
        # "#CSM \"Events: Unregister\"\nUnregister user event."
        n104 = Unregister For Events(event registration refnum=w271) -> (error out=w272:errorcluster)  [unwired: 1 in]
      }
      frame "---------- UI ----------" {
        # "#CSM \"Category Seperator\"\nDo not put any code in this frame."
        n105 = call <vilib>:"Add State(s) to Queue__JKI_lib_State_Machine.vi"("State(s) in (\"\")"=w278) -> ("States Out"=w277:string)  [unwired: 14 in]
      }
      frame "UI: Initialize" {
        w281 = "曲线编辑" ("前面板窗口:标题")
        w286 = u32 13816530
        # "树形清空"
        # "#CSM \"UI: Initialize\"\nInitialize the User Interface, here.\n(this is called automatically, by the Macro: Init)"
        n106 = control-ref of="循环树形"() -> (w287:refnum<vi>)
        n107 = control-ref of="循环树形"() -> (w295:refnum<vi>)
        n108 = control-ref of="窗格"() -> (w294:refnum<vi>)
        n109 = local write "总时长[秒]"(0.0 ("总时长[秒]")) -> ()
        n110 = control-ref of="动作列表框"() -> (w289:refnum<vi>)
        n111 = property class="Pane"(reference=w294, "Origin"=T4 {"Horizontal"=0, "Vertical"=0} ("原点")) -> ()  [unwired: 1 in, 2 out]
        n112 = property class="Tree (strict)"(reference=w295, "Allow Drop"=FALSE ("拖曳/放置:允许放置")) -> ()  [unwired: 1 in, 2 out]
        n113 = call "InitializeCurveList.vi"("循环树形"=w287, "ListBox输入"=w289) -> ("颜色符号列表"=w284:cluster{"项名":string, "颜色":u32, "符号":i32}[], "Tree引用输出"=w288:refnum<vi>)  [unwired: 6 in, 2 out]
        n114 = property class="Tree (strict)"(reference=w287, "SelColor"=w286) -> ()  [unwired: 1 in, 2 out]
        n115 = local write "曲线预览"(cluster{"X":dbl[], "Y":dbl[]} {"X"=[], "Y"=[]} ("曲线预览")) -> ()
        n116 = property on="动作列表框" class="LstBox (strict)"("SelColor"=w286) -> ()  [unwired: 2 in, 2 out]
        n117 = control-ref of="本VI"() -> (w282:refnum<vi>)
        n118 = invoke class="Tree (strict)" method="Edit Tree Items.Delete"(reference=w288) -> ()  [unwired: 4 in, 5 out]
        n119 = property class="VI"(reference=w282, "Front Panel.Title"=w281) -> (reference out=w279:refnum<vi>)  [unwired: 1 in, 1 out]
        n120 = Bundle By Name(cluster=w285, "User Data.颜色符号列表"=w284, "User Data.窗体标题"=w281) -> (w283:T9)
        n121 = control-ref of="Tab Control"() -> (w280:refnum<vi>)
        n122 = call "Match VI Window With TabControl.vi"("TabCtl Reference"=w280, "VI Reference"=w279) -> ()  [unwired: 10 in]
        n123 = call <vilib>:"Add State(s) to Queue__JKI_lib_State_Machine.vi"("State(s) in (\"\")"=w298) -> ("States Out"=w297:string)  [unwired: 14 in]
      }
      frame "UI: Cursor Set" {
        # "Argument"
        # "#CSM \"UI: Cursor Set\"\nSet and Unset Cursor Busy.\n(Usage: \"UI: Cursor Set >> Busy|Idle\")"
        n124 = disable-structure shown="TARGET_TYPE!=Windows" {
          disable-tunnel: [w306 _] -> w301
          disable-tunnel: w300 -> [w305 _]
          frame condition #0 (active) {
            n125 = case shown="\"Idle\", Default" w305 {
              tunnel: [w307 w308] -> w306
              frame "Idle", Default {
                n126 = call <vilib>:"Unset Busy.vi"() -> ("error out"=w307:errorcluster)  [unwired: 11 in]
              }
              frame "Busy" {
                n127 = call <vilib>:"Set Busy.vi"() -> ("error out"=w308:errorcluster)  [unwired: 10 in, 1 out]
              }
            }
          }
          frame condition #1 {
          }
        }
        n128 = call <vilib>:"Add State(s) to Queue__JKI_lib_State_Machine.vi"("State(s) in (\"\")"=w304) -> ("States Out"=w303:string)  [unwired: 14 in]
      }
      frame "UI: Front Panel State" {
        # "Argument"
        # "#CSM \"UI: Front Panel State\"\nSet Front Panel Open or Closed\n(Usage: \"UI: Front Panel State >> Open|Close\")"
        n129 = Unbundle By Name(w312) -> ("Core.Current VI Reference"=w311:refnum<vi>)
        n130 = case shown="\"Close\", \"Closed\"" w310 {
          tunnel: [w322 w335 w346 w358 w370] -> w313
          tunnel: w311 -> [w321 w333 w345 w357 w369]
          frame "Open", "Standard", Default {
            w316 = T1."Standard" ("State")
            n131 = property class="VI"(reference=w321) -> (reference out=w319:refnum<vi>, error out=w320:errorcluster, "FP.State"=w318:T1)  [unwired: 1 in]
            n132 = Not Equal?(x=w318, y=w316) -> (x != y?=w317:bool)
            n133 = case shown="True" w317 {
              tunnel: [w326 w328] -> w322
              tunnel: w320 -> [w325 w328]
              tunnel: w319 -> [w324 _]
              tunnel: w316 -> [w323 _]
              frame True {
                n134 = invoke class="VI" method="FP.Open"(reference=w324, error in=w325, "Activate"=TRUE, "State"=w323) -> (error out=w326:errorcluster)  [unwired: 1 in, 4 out]
              }
              frame False {
              }
            }
          }
          frame "Close", "Closed" {
            n135 = property class="VI"(reference=w333) -> (reference out=w332:refnum<vi>, error out=w334:errorcluster, "FP.State"=w330:T1)  [unwired: 1 in]
            n136 = Not Equal?(x=w330, y=T1."Closed" ("Front Panel Window:State")) -> (x != y?=w329:bool)
            n137 = case shown="True" w329 {
              tunnel: [w336 w339] -> w335
              tunnel: w334 -> [w336 w338]
              tunnel: w332 -> [_ w337]
              frame False {
              }
              frame True {
                n138 = invoke class="VI" method="FP.Close"(reference=w337, error in=w338) -> (error out=w339:errorcluster)  [unwired: 1 in, 2 out]
              }
            }
          }
          frame "Hidden", "Hide" {
            w340 = T1."Hidden" ("State")
            n139 = property class="VI"(reference=w345) -> (reference out=w343:refnum<vi>, error out=w344:errorcluster, "FP.State"=w342:T1)  [unwired: 1 in]
            n140 = Not Equal?(x=w342, y=w340) -> (x != y?=w341:bool)
            n141 = case shown="True" w341 {
              tunnel: [w350 w351] -> w346
              tunnel: w344 -> [w349 w351]
              tunnel: w343 -> [w348 _]
              tunnel: w340 -> [w347 _]
              frame True {
                n142 = invoke class="VI" method="FP.Open"(reference=w348, error in=w349, "State"=w347) -> (error out=w350:errorcluster)  [unwired: 2 in, 4 out]
              }
              frame False {
              }
            }
          }
          frame "Minimize", "Minimized" {
            w352 = T1."Minimized" ("State")
            n143 = property class="VI"(reference=w357) -> (reference out=w355:refnum<vi>, error out=w356:errorcluster, "FP.State"=w354:T1)  [unwired: 1 in]
            n144 = Not Equal?(x=w354, y=w352) -> (x != y?=w353:bool)
            n145 = case shown="False" w353 {
              tunnel: [w362 w363] -> w358
              tunnel: w356 -> [w361 w363]
              tunnel: w355 -> [w360 _]
              tunnel: w352 -> [w359 _]
              frame True {
                n146 = invoke class="VI" method="FP.Open"(reference=w360, error in=w361, "State"=w359) -> (error out=w362:errorcluster)  [unwired: 2 in, 4 out]
              }
              frame False {
              }
            }
          }
          frame "Maximize", "Maximized" {
            w364 = T1."Maximized" ("State")
            n147 = property class="VI"(reference=w369) -> (reference out=w367:refnum<vi>, error out=w368:errorcluster, "FP.State"=w366:T1)  [unwired: 1 in]
            n148 = Not Equal?(x=w366, y=w364) -> (x != y?=w365:bool)
            n149 = case shown="True" w365 {
              tunnel: [w374 w375] -> w370
              tunnel: w368 -> [w373 w375]
              tunnel: w367 -> [w372 _]
              tunnel: w364 -> [w371 _]
              frame True {
                n150 = invoke class="VI" method="FP.Open"(reference=w372, error in=w373, "State"=w371) -> (error out=w374:errorcluster)  [unwired: 2 in, 4 out]
              }
              frame False {
              }
            }
          }
        }
        n151 = call <vilib>:"Add State(s) to Queue__JKI_lib_State_Machine.vi"("State(s) in (\"\")"=w315) -> ("States Out"=w314:string)  [unwired: 14 in]
      }
      frame "---------- Macro ----------" {
        # "#CSM \"Category Seperator\"\nDo not put any code in this frame."
        n152 = call <vilib>:"Add State(s) to Queue__JKI_lib_State_Machine.vi"("State(s) in (\"\")"=w379) -> ("States Out"=w378:string)  [unwired: 14 in]
      }
      frame "Macro: Initialize" {
        w381 = "Data: Initialize\nInitialize Core Data\nEvents: Register\nUI: Initialize\nUI: Front Panel State >> Open"  # Data: Initialize Initialize Core Data Events: Register UI: Initialize UI: Front Panel State >> Open
        # "#CSM \"Macro: Initialize\"\nInitialization Macro (This is called once, when the VI starts)"
        n153 = call <vilib>:"Add State(s) to Queue__JKI_lib_State_Machine.vi"("State(s) in Front (\"\")"=w381, "State(s) in (\"\")"=w384) -> ("States Out"=w383:string)  [unwired: 13 in]
      }
      frame "Macro: Exit" {
        # "#CSM \"Macro: Exit\"\nExit Macro (This is called once, when the VI exits)"
        n154 = Unbundle By Name(w393) -> ("Core.Close Panel on Exit?"=w392:bool)
        n155 = Select(t="UI: Front Panel State >> Close", s=w392, f="") -> (s? t:f=w389:string)
        n156 = call <vilib>:"Add State(s) to Queue__JKI_lib_State_Machine.vi"("State(s) in Front (\"\")"="//Exit Sub-Modules ", "State(s) in (\"\")"=w389, "State(s) at Back (\"\")"="Data: Cleanup\nEvents: Unregister\nExit") -> ("States Out"=w387:string)  [unwired: 12 in]
        n157 = call <vilib>:"Add State(s) to Queue__JKI_lib_State_Machine.vi"("State(s) in Front (\"\")"=w387, "State(s) in (\"\")"=w395) -> ("States Out"=w394:string)  [unwired: 13 in]
      }
      frame "---------- API ----------" {
        # "#CSM \"Category Seperator\"\nDo not put any code in this frame."
      }
      frame "---------- Action ----------" {
        # "#CSM \"Category Seperator\"\nDo not put any code in this frame."
        n158 = call <vilib>:"Add State(s) to Queue__JKI_lib_State_Machine.vi"("State(s) in (\"\")"=w402) -> ("States Out"=w401:string)  [unwired: 14 in]
      }
      frame "Action: Write File" {
        # "#CSM \"Internal State\"\nThis category is used for holding internal states"
        n159 = Unbundle By Name(w403) -> ("User Data.存盘提醒"=w405:bool, "User Data.文件路径"=w407:path, "User Data.窗体标题"=w406:string, "User Data.循环数组"=w408:string[])
        n160 = for {
          tunnel: w408 -> [w438] mode=indexing
          shift-right: [w435] -> w414
          shift-left: "" -> [w436]
          i -> [w443]
          # "将字符串数组转换为换行符分隔的字符串"
          n161 = Equal To 0?(x=w443) -> (x = 0?=w442:bool)
          n162 = Select(t="", s=w442, f="\n") -> (s? t:f=w439:string)
          n163 = Concatenate Strings(w439, w438) -> (w437:string)
          n164 = Concatenate Strings(w436, w437) -> (w435:string)
        }
        n165 = Open/Create/Replace File(file path (use dialog)=w407, operation (0:open)=T5."replace or create" ("操作(0:open)"), access (0:read/write)=enum16{"read/write", "read-only", "write-only"}."write-only" ("权限(0:read/write)")) -> (refnum out=w411:refnum<file>, error out=w412:errorcluster)  [unwired: 3 in, 1 out]
        n166 = Write to Text File(file (use dialog)=w411, text=w414, error in=w412) -> (refnum out=w415:refnum<file>, error out=w416:errorcluster)  [unwired: 1 in, 1 out]
        n167 = Close File(refnum=w415, error in=w416) -> (path=w418:path, error out=w417:errorcluster)
        n168 = case shown="No Error" w417 {
          tunnel: w418 -> [w427 _]
          tunnel: w406 -> [w426 _]
          tunnel: w405 -> [w425 _]
          tunnel: w403 -> [w424 w433]
          tunnel: [w422 w433] -> w404
          frame No Error {
            n169 = call <vilib>:"Get File Extension.vi"("file"=w427) -> ("filename without extension"=w429:string)  [unwired: 6 in, 4 out]
            n170 = Bundle By Name(cluster=w424, "User Data.文件已保存"=TRUE ("文件已保存")) -> (w422:T9)
            n171 = case shown="True" w425 {
              frame False {
              }
              frame True {
                n172 = One Button Dialog(message="文件保存成功！" ("消息")) -> ()  [unwired: 1 in, 1 out]
              }
            }
            n173 = control-ref of="本VI"() -> (w428:refnum<vi>)
            n174 = Concatenate Strings(w429, " - " ("字符串"), w426) -> (w431:string)
            n175 = property class="VI"(reference=w428, "Front Panel.Title"=w431) -> ()  [unwired: 1 in, 2 out]
          }
          frame Error {
            n176 = One Button Dialog(message="文件保存失败！" ("消息")) -> ()  [unwired: 1 in, 1 out]
          }
        }
        n177 = call <vilib>:"Add State(s) to Queue__JKI_lib_State_Machine.vi"("State(s) in (\"\")"=w421) -> ("States Out"=w420:string)  [unwired: 14 in]
      }
      frame "Action: Read File" {
        # "#CSM \"Internal State\"\nThis category is used for holding internal states"
        n178 = Unbundle By Name(w447) -> ("User Data.文件路径"=w451:path, "User Data.颜色符号列表"=w450:cluster{"项名":string, "颜色":u32, "符号":i32}[], "User Data.窗体标题"=w449:string)
        n179 = call-poly <vilib>:"Read Delimited Spreadsheet.vi"("file path (dialog if empty)"=w451) -> ("all rows"=w446:string[][])  [unwired: 9 in, 5 out]
        n180 = Index Array(array=w446, index (col)=0 ("禁用的索引 (列)")) -> (element=w454:string[])  [unwired: 1 in]
        n181 = control-ref of="循环树形"() -> (w453:refnum<vi>)
        n182 = call "Array2Tree.vi"("颜色符号列表"=w450, "循环数组"=w454, "循环树形引用输入"=w453) -> ("错误输出"=w455:errorcluster, "循环树形引用输出"=w456:refnum<vi>)  [unwired: 7 in]
        n183 = case shown="No Error" w455 {
          tunnel: w451 -> [w459 _]
          tunnel: w456 -> [w467 _]
          tunnel: w449 -> [w466 _]
          tunnel: w447 -> [w465 w473]
          tunnel: [w462 w473] -> w448
          tunnel: w445 -> [w461 w472]
          tunnel: [w460 w472] -> w444
          frame No Error {
            n184 = call <vilib>:"Get File Extension.vi"("file"=w459) -> ("filename without extension"=w469:string)  [unwired: 6 in, 4 out]
            n185 = call "Tree2Array.vi"("TreeControl输入"=w467) -> ("循环数组"=w463:string[])  [unwired: 9 in, 1 out]
            n186 = Bundle By Name(cluster=w465, "User Data.文件已保存"=TRUE ("文件已保存"), "User Data.循环数组"=w463) -> (w462:T9)
            n187 = control-ref of="本VI"() -> (w468:refnum<vi>)
            n188 = call <vilib>:"Add State(s) to Queue__JKI_lib_State_Machine.vi"("State(s) in (\"\")"=w461, "State(s) at Back (\"\")"="Action: Draw Plot" ("State(s) at Back (\"\")")) -> ("States Out"=w460:string)  [unwired: 13 in]
            n189 = Concatenate Strings(w469, " - " ("字符串"), w466) -> (w471:string)
            n190 = property class="VI"(reference=w468, "Front Panel.Title"=w471) -> ()  [unwired: 1 in, 2 out]
          }
          frame Error {
          }
        }
      }
      frame "Action: Draw Plot" {
        n191 = Unbundle By Name(w475) -> ("User Data.循环数组"=w474:string[])
        n192 = call "DrawCurve.vi"("曲线定义数组"=w474) -> ("曲线输出"=w480:cluster{"X":dbl[], "Y":dbl[]})  [unwired: 10 in]
        "曲线预览" <- w480
        n193 = Unbundle(w480) -> ("X"=w479:dbl[])  [unwired: 1 out]
        n194 = Delete From Array(array=w479, length=1 ("长度")) -> (deleted portion=w478:dbl[])  [unwired: 1 in, 1 out]
        n195 = Index Array(array=w478) -> (element=→"总时长[秒]":dbl)  [unwired: 1 in]
      }
      frame "Action: Handle Unsaved Porcess" {
        n196 = Two Button Dialog(message="是否保存现有文件？" ("消息"), 1:"不保存" ("F按钮名称（“取消”）"), 2:"保存" ("T按钮名称（“确定”）")) -> (T button?=w491:bool)
        n197 = case shown="True" w491 {
          tunnel: [w495 w501] -> w487
          tunnel: w486 -> [w496 w502]
          tunnel: [w497 w500] -> w485
          tunnel: w484 -> [w497 w499]
          frame False {
            n198 = Bundle By Name(cluster=w496, "User Data.文件已保存"=TRUE ("新建按钮")) -> (w495:T9)
          }
          frame True {
            # "文件要保存"
            n199 = Unbundle By Name(w502) -> ("User Data.文件路径"=w503:path, "User Data.文件参数"=w498:T11)
            n200 = control-ref of="本VI"() -> (w506:refnum<vi>)
            n201 = call "SaveFileDialogue.vi"("文件参数"=w498, "文件路径"=w503, "VI输入"=w506) -> ("错误输出"=w505:errorcluster, "输出路径"=w504:path)  [unwired: 6 in, 1 out]
            n202 = case shown="No Error" w505 {
              tunnel: w504 -> [w513 _]
              tunnel: [w510 w516] -> w501
              tunnel: w502 -> [w514 w516]
              tunnel: [w508 w515] -> w500
              tunnel: w499 -> [w509 w515]
              frame No Error {
                n203 = control-ref of="循环树形"() -> (w512:refnum<vi>)
                n204 = call "Tree2Array.vi"("TreeControl输入"=w512) -> ("循环数组"=w511:string[])  [unwired: 9 in, 1 out]
                n205 = Bundle By Name(cluster=w514, "User Data.文件路径"=w513, "User Data.循环数组"=w511) -> (w510:T9)
                n206 = call <vilib>:"Add State(s) to Queue__JKI_lib_State_Machine.vi"("State(s) in Front (\"\")"="Action: Write File" ("State(s) in Front (\"\")"), "State(s) in (\"\")"=w509) -> ("States Out"=w508:string)  [unwired: 13 in]
              }
              frame Error {
              }
            }
          }
        }
      }
      frame "Action: Open File" {
        n207 = Unbundle By Name(w520) -> ("User Data.文件参数"=w521:T11)
        n208 = Unbundle By Name(w521) -> ("默认路径"=w524:path, "类型(后缀名)"=w523:string, "类型标签"=w522:string)
        n209 = call "文件对话框"("start path"=w524, "pattern (all files)"=w523, "pattern label"=w522) -> ("selected path"=w525:path, "exists"=w527:bool, "error out"=w526:errorcluster)  [unwired: 9 in, 1 out]
        n210 = case shown="No Error" w526 {
          tunnel: w525 -> [w534 _]
          tunnel: w527 -> [w535 _]
          tunnel: w520 -> [w532 w545]
          tunnel: w519 -> [w530 w544]
          tunnel: [w533 w545] -> w518
          tunnel: [w531 w544] -> w517
          frame No Error {
            n211 = case shown="True" w535 {
              tunnel: w534 -> [_ w541]
              tunnel: [w537 w542] -> w533
              tunnel: w532 -> [w537 w543]
              tunnel: [w536 w539] -> w531
              tunnel: w530 -> [w536 w540]
              frame False {
              }
              frame True {
                n212 = Bundle By Name(cluster=w543, "User Data.文件路径"=w541) -> (w542:T9)
                n213 = call <vilib>:"Add State(s) to Queue__JKI_lib_State_Machine.vi"("State(s) in (\"\")"=w540, "State(s) at Back (\"\")"="Action: Read File" ("State(s) at Back (\"\")")) -> ("States Out"=w539:string)  [unwired: 13 in]
              }
            }
          }
          frame Error {
          }
        }
      }
      frame "Action: Save File" {
        n214 = Unbundle By Name(w550) -> ("User Data.文件参数"=w549:T11)
        n215 = call "Convert API String Arguments to Data.vim"("Reference Type"=path "", "API String"=w548) -> ("Data"=w547:path)  [unwired: 6 in, 1 out]
        n216 = control-ref of="本VI"() -> (w554:refnum<vi>)
        n217 = call "SaveFileDialogue.vi"("文件参数"=w549, "文件路径"=w547, "VI输入"=w554) -> ("错误输出"=w556:errorcluster, "输出路径"=w555:path)  [unwired: 6 in, 1 out]
        n218 = case shown="No Error" w556 {
          tunnel: w555 -> [w563 _]
          tunnel: w550 -> [w565 w568]
          tunnel: [w564 w568] -> w553
          tunnel: [w561 w567] -> w552
          tunnel: w551 -> [w560 w567]
          frame No Error {
            n219 = control-ref of="循环树形"() -> (w566:refnum<vi>)
            n220 = call "Tree2Array.vi"("TreeControl输入"=w566) -> ("循环数组"=w562:string[])  [unwired: 9 in, 1 out]
            n221 = Bundle By Name(cluster=w565, "User Data.文件路径"=w563, "User Data.循环数组"=w562) -> (w564:T9)
            n222 = call <vilib>:"Add State(s) to Queue__JKI_lib_State_Machine.vi"("State(s) in (\"\")"=w560, "State(s) at Back (\"\")"="Action: Write File" ("State(s) at Back (\"\")")) -> ("States Out"=w561:string)  [unwired: 13 in]
          }
          frame Error {
          }
        }
      }
      frame "Action: New File" {
        w576 = "曲线" ("左单元格字符串")
        n223 = Unbundle By Name(w571) -> ("User Data.文件参数"=w570:T11, "User Data.窗体标题"=w569:string)
        n224 = control-ref of="循环树形"() -> (w587:refnum<vi>)
        n225 = control-ref of="本VI"() -> (w586:refnum<vi>)
        n226 = local write "总时长[秒]"(0.0 ("总时长[秒]")) -> ()
        n227 = invoke class="Tree (strict)" method="Edit Tree Items.Delete"(reference=w587) -> (reference out=w583:refnum<vi>)  [unwired: 4 in, 4 out]
        n228 = local write "曲线预览"(cluster{"X":dbl[], "Y":dbl[]} {"X"=[], "Y"=[]} ("曲线预览")) -> ()
        n229 = Unbundle By Name(w570) -> ("默认名称"=w584:string)
        n230 = Concatenate Strings(w584, " - " ("字符串"), w569) -> (w585:string)
        n231 = property class="VI"(reference=w586, "Front Panel.Title"=w585) -> ()  [unwired: 1 in, 2 out]
        n232 = invoke class="Tree (strict)" method="Edit Tree Items.Add Item"(reference=w583, "Child Position"=-1 ("子项位置"), "Left Cell"=w576, "Child Tag"=w576) -> (reference out=w582:refnum<vi>, "Edit Tree Items:Add Item"=w581:string)  [unwired: 5 in, 7 out]
        n233 = call "Tree2Array.vi"("TreeControl输入"=w582) -> ("循环数组"=w572:string[])  [unwired: 9 in, 1 out]
        n234 = property class="Tree (strict)"(reference=w582, "Active Item Tag"=w581, "Glyph"=1 ("活动项:符号索引")) -> ()  [unwired: 1 in, 2 out]
        n235 = Bundle By Name(cluster=w571, "User Data.文件路径"=path "", "User Data.循环数组"=w572) -> (w574:T9)
        n236 = call <vilib>:"Add State(s) to Queue__JKI_lib_State_Machine.vi"("State(s) in (\"\")"=w590) -> ("States Out"=w589:string)  [unwired: 14 in]
      }
      frame "Action: Edit Item" {
        # "通过标识获取行索引和首列文本"
        n237 = control-ref of="循环树形"() -> (w596:refnum<vi>)
        n238 = property class="Tree (strict)"(reference=w596, "ActiveColNum"=0 ("活动单元格:活动列数")) -> (reference out=w599:refnum<vi>, error out=w598:errorcluster, "Active Item Row Number"=w600:i32, "Indent Level"=w601:i32, "Cell String"=w597:string)  [unwired: 1 in]
        n239 = case shown="No Error" w598 {
          selector: w598 -> [_ w633]
          tunnel: w597 -> [w612 _]
          tunnel: w599 -> [w611 _]
          tunnel: w600 -> [w610 _]
          tunnel: w601 -> [w609 _]
          tunnel: [w607 w632] -> w594
          tunnel: w593 -> [w606 w632]
          tunnel: [w605 w631] -> w592
          tunnel: w591 -> [w604 w631]
          frame No Error {
            n240 = Not Equal To 0?(x=w609) -> (x != 0?=w608:bool)
            n241 = case shown="True" w608 {
              tunnel: w612 -> [_ w626]
              tunnel: w611 -> [_ w625]
              tunnel: w610 -> [_ w622]
              tunnel: [w614 w620] -> w607
              tunnel: w606 -> [w614 w621]
              tunnel: [w613 w617] -> w605
              tunnel: w604 -> [w613 w616]
              frame False {
              }
              frame True {
                # "编辑窗打开，文件变为未保存"
                # "打开编辑窗口"
                # "动作选择"
                # "当为子项时打开编辑窗口"
                n242 = case shown="\"抛物线\"" w626 {
                  tunnel: [w627 w628 w629 w630] -> w623
                  frame "假", Default {
                    n243 = vi-ref "EditLine.vi"() -> (w627:refnum<vi>)
                  }
                  frame "直线" {
                    n244 = vi-ref "EditLine.vi"() -> (w628:refnum<vi>)
                  }
                  frame "正弦" {
                    n245 = vi-ref "EditSine.vi"() -> (w629:refnum<vi>)
                  }
                  frame "抛物线" {
                    n246 = vi-ref "EditParabola.vi"() -> (w630:refnum<vi>)
                  }
                }
                n247 = call "CallEditVI.vi"("VI引用句柄"=w623, "索引"=w622, "TreeControl输入"=w625) -> ("TreeControl输出"=w624:refnum<vi>)  [unwired: 7 in, 1 out]
                n248 = call "Tree2Array.vi"("TreeControl输入"=w624) -> ("循环数组"=w619:string[])  [unwired: 9 in, 1 out]
                n249 = Bundle By Name(cluster=w621, "User Data.循环数组"=w619, "User Data.文件已保存"=FALSE ("文件已保存")) -> (w620:T9)
                n250 = call <vilib>:"Add State(s) to Queue__jki_lib_state_machine.vi"("State(s) in (\"\")"=w616, "State(s) at Back (\"\")"="Action: Draw Plot" ("State(s) at Back (\"\")")) -> ("States Out"=w617:string)  [unwired: 13 in]
              }
            }
          }
          frame Error {
            n251 = call <vilib>:"Clear Errors.vi"("error in (no error)"=w633) -> ()  [unwired: 5 in, 2 out]
          }
        }
      }
    }
  }
